vi "MoD Main-Optimize - HPLC - SUZUKI 04122017_ Simulate.vi"() -> ()   [LabVIEW 2015]
uses:
  <vilib>/ni845x/ni845x.llb/ni845xControl.ctl
  <vilib>/addons/control/pid/pid.llb/PID Control Input Filter (DBL).vi
  <vilib>/addons/control/pid/autopid.llb/PID Online Autotuning (Relay Feedback).vi
  <vilib>/addons/control/pid/NI_PID_autopid.lvlib
  <vilib>/addons/control/pid/NI_PID_pid.lvlib
  <vilib>/MakerHub/LINX/LMH-LINX.lvlib
  <vilib>/MakerHub/LINX/Public/Peripherals/Digital/Digital Write 1 Chan.vi
panel:
  out "Is current Exp a Redo?":bool=TRUE
  in  "Debug_run_button":bool
  out "Phase_Sensor_voltage":dbl
  out "P_tot":dbl
  out "pause for ms":bool=TRUE
  out "stop_xl_write":bool=TRUE
  out "Num_exp_till_pause":i32
  out "Syringe_pump?":bool=TRUE
  out "System Error":bool=TRUE
  out "error out":errorcluster
  out "Pump setpoint(ul/min) 6":dbl format="%#_13g"
  out "Pump setpoint(ul/min) 5":dbl format="%#_13g"
  out "Pump setpoint(ul/min) 4":dbl format="%#_13g"
  out "Pump setpoint(ul/min) 3":dbl format="%#_13g"
  out "Pump setpoint(ul/min) 2":dbl format="%#_13g"
  out "Pump setpoint(ul/min) 1":dbl format="%#_13g"
  out "Volume (ul) 5":dbl format="%#_13g"
  out "Volume (ul) 4":dbl format="%#_13g"
  out "Volume (ul) 3":dbl format="%#_13g"
  out "Volume (ul) 2":dbl format="%#_13g"
  out "Volume (ul) 1":dbl format="%#_13g"
  in  "tau 5":dbl format="%#_13g"
  out "tau 4":dbl format="%#_13g"
  out "tau 3":dbl format="%#_13g"
  out "tau 2":dbl format="%#_13g"
  out "tau 1":dbl format="%#_13g"
  out "Reactor Length":dbl format="%#_13g"
  out "Flowrate Sensor 2":dbl format="%#_13g"
  out "Flowrate Sensor 1":dbl format="%#_13g"
  out "Pressure 2":dbl format="%#_13g"
  out "Pressure 1":dbl format="%#_13g"
  out "Temperature Control 5":bool=TRUE
  out "Temperature Control 4":bool=TRUE
  out "Temperature Control 3":bool=TRUE
  out "Temperature Control 2":bool=TRUE
  out "Temperature Control 1":bool=TRUE
  out "Temperature SP 5":dbl format="%#_g'C"
  out "Temperature SP 4":dbl format="%#_g'C"
  out "Temperature SP 3":dbl format="%#_g'C"
  out "Temperature SP 2":dbl format="%#_g'C"
  out "Temperature SP 1":dbl format="%#_g'C"
  in  "Bay Temperature 5":dbl
  in  "SSR Duration 5":dbl
  in  "SSR Duration 4":dbl
  in  "SSR Duration 3":dbl
  in  "SSR Duration 2":dbl
  in  "SSR Duration 1":dbl
  in  "Total Product Amount":dbl=1.0 format="%#_gml"
  out "Setup Error":bool=TRUE
  out "Error Message":string
  out "ID CTR":i32
  in  "Tab Control 2":enum32{"Faults", "Devices"}(tab)=enum."Devices"
  out "Fault Cluster":T1
  in  "COMM Port:: Harvard Syringe Pump":refnum<visa-resource-name>="COM5"
  in  "Sample Valve COMM::Port":refnum<visa-resource-name>="COM6"
  in  "Arduino COMM Port":refnum<visa-resource-name>="COM3"
  in  "COMM Port :: Milligat Pumps":refnum<visa-resource-name>="COM10"
  in  "IR Sensor Device":T2="USB0::0x3923::0x7514::01B3FF21::RAW"
  in  "Tab Control":enum32{"Setup", "Parameters", "Monitoring"}(tab)
  in  "System decide help Button":bool
  in  "Reaction Scheme Confirm":bool
  in  "Synthesis Route Array":string[](array[string])=["3-Br-Pyridine _ Biphenyl", "K2CO3", "PhB(OH)2", "", "", ""]
  in  "Manual/Automated":bool
  in  "Save Button":bool
  in  "Open Button":bool
  in  "New rxn scheme button":bool
  in  "System decide help Button 2":bool
  out "Setup Confirm":bool=TRUE
  in  "BAY 1":u16(ring) items=["                 Bypass", "             Hot Reactor", "               Separator"]
  in  "BAY 5":u16(ring) items=["                     Bypass", "                Hot Reactor", "                 Separator"]
  in  "BAY 4":u16(ring) items=["                     Bypass", "                Hot Reactor", "                  Separator"]
  in  "BAY 3":u16(ring)=1 items=["                     Bypass", "                 Hot Reactor", "                  Separator"]
  in  "BAY 2":u16(ring) items=["                     Bypass", "                Hot Reactor", "                  Separator"]
  in  "System Parameters Help Button":bool
  in  "System Parameters Confirm Button":bool
  in  "Bay Parameters":T3={"Pump 1 Reagent Concentration"=0.8, "Pump 2 Reagent Concentration"=0.55, "Pump 3 Reagent Concentration"=0.4, "Pump 4 Reagent Concentration"=0.0, "Pump 5 Reagent Concentration"=0.0, "Bay 1 Parameters"={"Pump 1 Flowrate"=0.0, "optimize_temp"=FALSE, "optimize_tau"=TRUE, "Run at set flowrate"=FALSE, "Pump 2 Flowrate"=0.0, "Temperature Params"=[0.0, 40.0, 100.0], "pump params 1"=[0.0, 32.5, 325.0], "pump params 2"=[0.0, 32.5, 325.0]}, "Bay 2 Parameters"={"Pump 3 Flowrate"=0.0, "optimize_temp"=FALSE, "optimize_tau"=TRUE, "Run at set flowrate"=FALSE, "Temperature Params"=[0.0, 40.0, 100.0], "Resisdence time params"=[0.0, 65.0, 650.0], "pump_at_ratio"=FALSE, "pump_num_ratio"=0.0}, "Bay 3 Parameters"={"Pump 4 Flowrate"=0.0, "optimize_temp"=TRUE, "optimize_tau"=FALSE, "Run at set flowrate"=FALSE, "Temperature Params"=[0.0, 40.0, 100.0], "Resisdence time params"=[0.0, 0.0, 0.0], "pump_at_ratio"=FALSE, "pump_num_ratio"=0.0}, "Bay 4 Parameters"={"Pump 5 Flowrate"=40.0, "Run at set flowrate"=FALSE, "optimize_temp"=FALSE, "optimize_tau"=FALSE, "Resisdence time params"=[0.0, 36.0, 225.0], "Temperature Params"=[0.0, 40.0, 80.0], "pump_at_ratio"=FALSE, "pump_num_ratio"=0.0}, "Bay 5 Parameters"={"Pump 6 Flowrate"=0.0, "Run at set flowrate"=FALSE, "optimize_temp"=FALSE, "optimize_tau"=FALSE, "Resisdence time params"=[0.0, 0.0, 0.0], "Temperature Params"=[0.0, 0.0, 0.0], "pump_at_ratio"=FALSE, "pump_num_ratio"=0.2}, "Bay 1 Flow Rate Ratio \n(Pump 1: Pump 2)"=1.0, "tube_id(in)"=[enum.".02", enum.".03", enum.".03", enum.".03", enum.".03"], "xml_filename"="temp_xml", "Excel File Name"="C:\\Users\\HPLC\\Dropbox (MIT)\\MoD Files\\Data\\HWE Results\\SUZUKI Optimization HPLC - 04122017", "hplc File Name"="C:\\Chem32\\1\\Data\\MOD", "Matlab File"="C:\\Users\\HPLC\\Dropbox (MIT)\\MoD Files\\Data\\SUZUKI 04132017b", "Syringe for Pump 2?"=FALSE, "Num_conditons_per_wait"=1.0, "Continue from previous optimization?"=FALSE, "Pump 6 Reagent Concentration"=0.0, "Pause before analysis?"=FALSE, "Hplc Wait time(min)"=0.04} {"Hplc Wait time(min)" format="%#_13g"; "Pump 6 Reagent Concentration" format="%#_6gM"; "Bay 5 Parameters"."Temperature Params" format="%#_g'C"; "Bay 4 Parameters"."Temperature Params" format="%#_g'C"; "Bay 3 Parameters"."Temperature Params" format="%#_g'C"; "Bay 2 Parameters"."Temperature Params" format="%#_g'C"; "Bay 1 Parameters"."Temperature Params" format="%#_g'C"; "Pump 5 Reagent Concentration" format="%#_6gM"; "Pump 4 Reagent Concentration" format="%#_6gM"; "Pump 3 Reagent Concentration" format="%#_6gM"; "Pump 2 Reagent Concentration" format="%#_6gM"; "Pump 1 Reagent Concentration" format="%#_6gM"}
  out "System Confirm Not Clicked":string
  out "Setup Confirm 2":bool=TRUE
  out "Current Experiment":dbl
  in  "Total Number of Experiments":dbl=33.0
  out "Phase Sensor Chart":T4(graph)
  out "HPLC Analysis":bool
  out "Equlibrating Temperature":bool
  out "Flushing System":bool
  out "Calculate condition":bool
  out "System Flush Wait Time":u8(slide) scale=0.0..1149.042355163602
  out "Temperature 5":dbl format="%#_g'C"
  out "Temperature 4":dbl format="%#_g'C"
  out "Temperature 3":dbl format="%#_g'C"
  out "Temperature 2":dbl format="%#_g'C"
  out "Temperature 1":dbl format="%#_g'C"
  out "Flowrate Chart":T5(graph)
  out "Bay 5":u16(ring) items=["                     Bypass", "                   Reactor1", "               Separator"]
  out "Bay 4":u16(ring) items=["                     Bypass", "                   Reactor1", "               Separator"]
  out "Bay 3":u16(ring) items=["                     Bypass", "                   Reactor1", "               Separator"]
  out "Bay 2":u16(ring) items=["                     Bypass", "                   Reactor1", "               Separator"]
  out "Bay 1":u16(ring) items=["                     Bypass", "                   Reactor1", "               Separator"]
  out "Teperature Chart":T5(graph)
  out "Pump Setpoints Chart":T5(graph)
  out "Pressure Chart":T5(graph)
  out "Optimization_loop_index":i32
  out "curr_wait_time":dbl
  out "total_flush_time":dbl
  out "Temp SS? 5":bool=TRUE
  out "Temp SS? 4":bool=TRUE
  out "Temp SS? 3":bool=TRUE
  out "Temp SS? 2":bool=TRUE
  out "Temp SS? 1":bool=TRUE
  out "System Flushed?":bool
  out "stop_button clicked":bool
  out "Total System Resisdence Time(min)":dbl
  out "Will Redo Next Exp?":bool=TRUE
  out "Stop":bool=TRUE
  in  "Run_Stop_cluster":T6
  # "Molecules on Demand"
  # "Synthesis Route"
  # "Reagent List"
  # "1"
  # "2"
  # "1"
  # "3"
  # "2"
  # "4"
  # "3"
  # "5"
  # "4"
  # "6"
  # "5"
  # "Product"
  # "6"
  # "Have system decide based on synthesis route"
  # "Manually enter bay configuration"
  # "System Schematic"
  # "Optimization Parameters"
  # "Bay"
  # "Tube ID (in)"
  # "1."
  # "2."
  # "3."
  # "4."
  # "5."
  # "Pause after"
  # "Experiments"
  # "Reporting"
  # "XML Output File Name"
  # "Excel Output File Name"
  # "HPLC File Path"
  # "MATLAB File Path"
  # "Temperature"
  # "Flowrate(ul/min)"
  # "Setpoint"
  # "Lower Bound"
  # "Upper Bound"
  # "Optimize?"
  # "-or-"
  # "Run at"
  # "times incoming flow"
  # "Temperature"
  # "Flowrate(ul/min)"
  # "Setpoint"
  # "Lower Bound"
  # "Upper Bound"
  # "Optimize?"
  # "-or-"
  # "Run at"
  # "times incoming flow"
  # "Temperature"
  # "Flowrate(ul/min)"
  # "Setpoint"
  # "Lower Bound"
  # "Upper Bound"
  # "Optimize?"
  # "-or-"
  # "Run at"
  # "times incoming flow"
  # "Temperature"
  # "Flowrate 3 (ul/min)"
  # "Setpoint"
  # "Lower Bound"
  # "Upper Bound"
  # "Optimize?"
  # "-or-"
  # "Run at"
  # "times incoming flow"
  # "Temperature"
  # "Flowrate 1(ul/min)"
  # "Flowrate 2(ul/min)"
  # "Setpoint"
  # "Lower Bound"
  # "Upper Bound"
  # "Optimize?"
  # "Temperature('C)"
  # "Pressure (psi)"
  # "Flowrate (ul/min)"
  # "Pump Flowrate Setpoints(ul/min)"
  # "Phase Sensor Value"
  # "Experimental Steps"
  # "Calculated new conditions"
  # "Flushed System"
  # "Analyzed HPLC"
  # "Equilibrated Temperature"
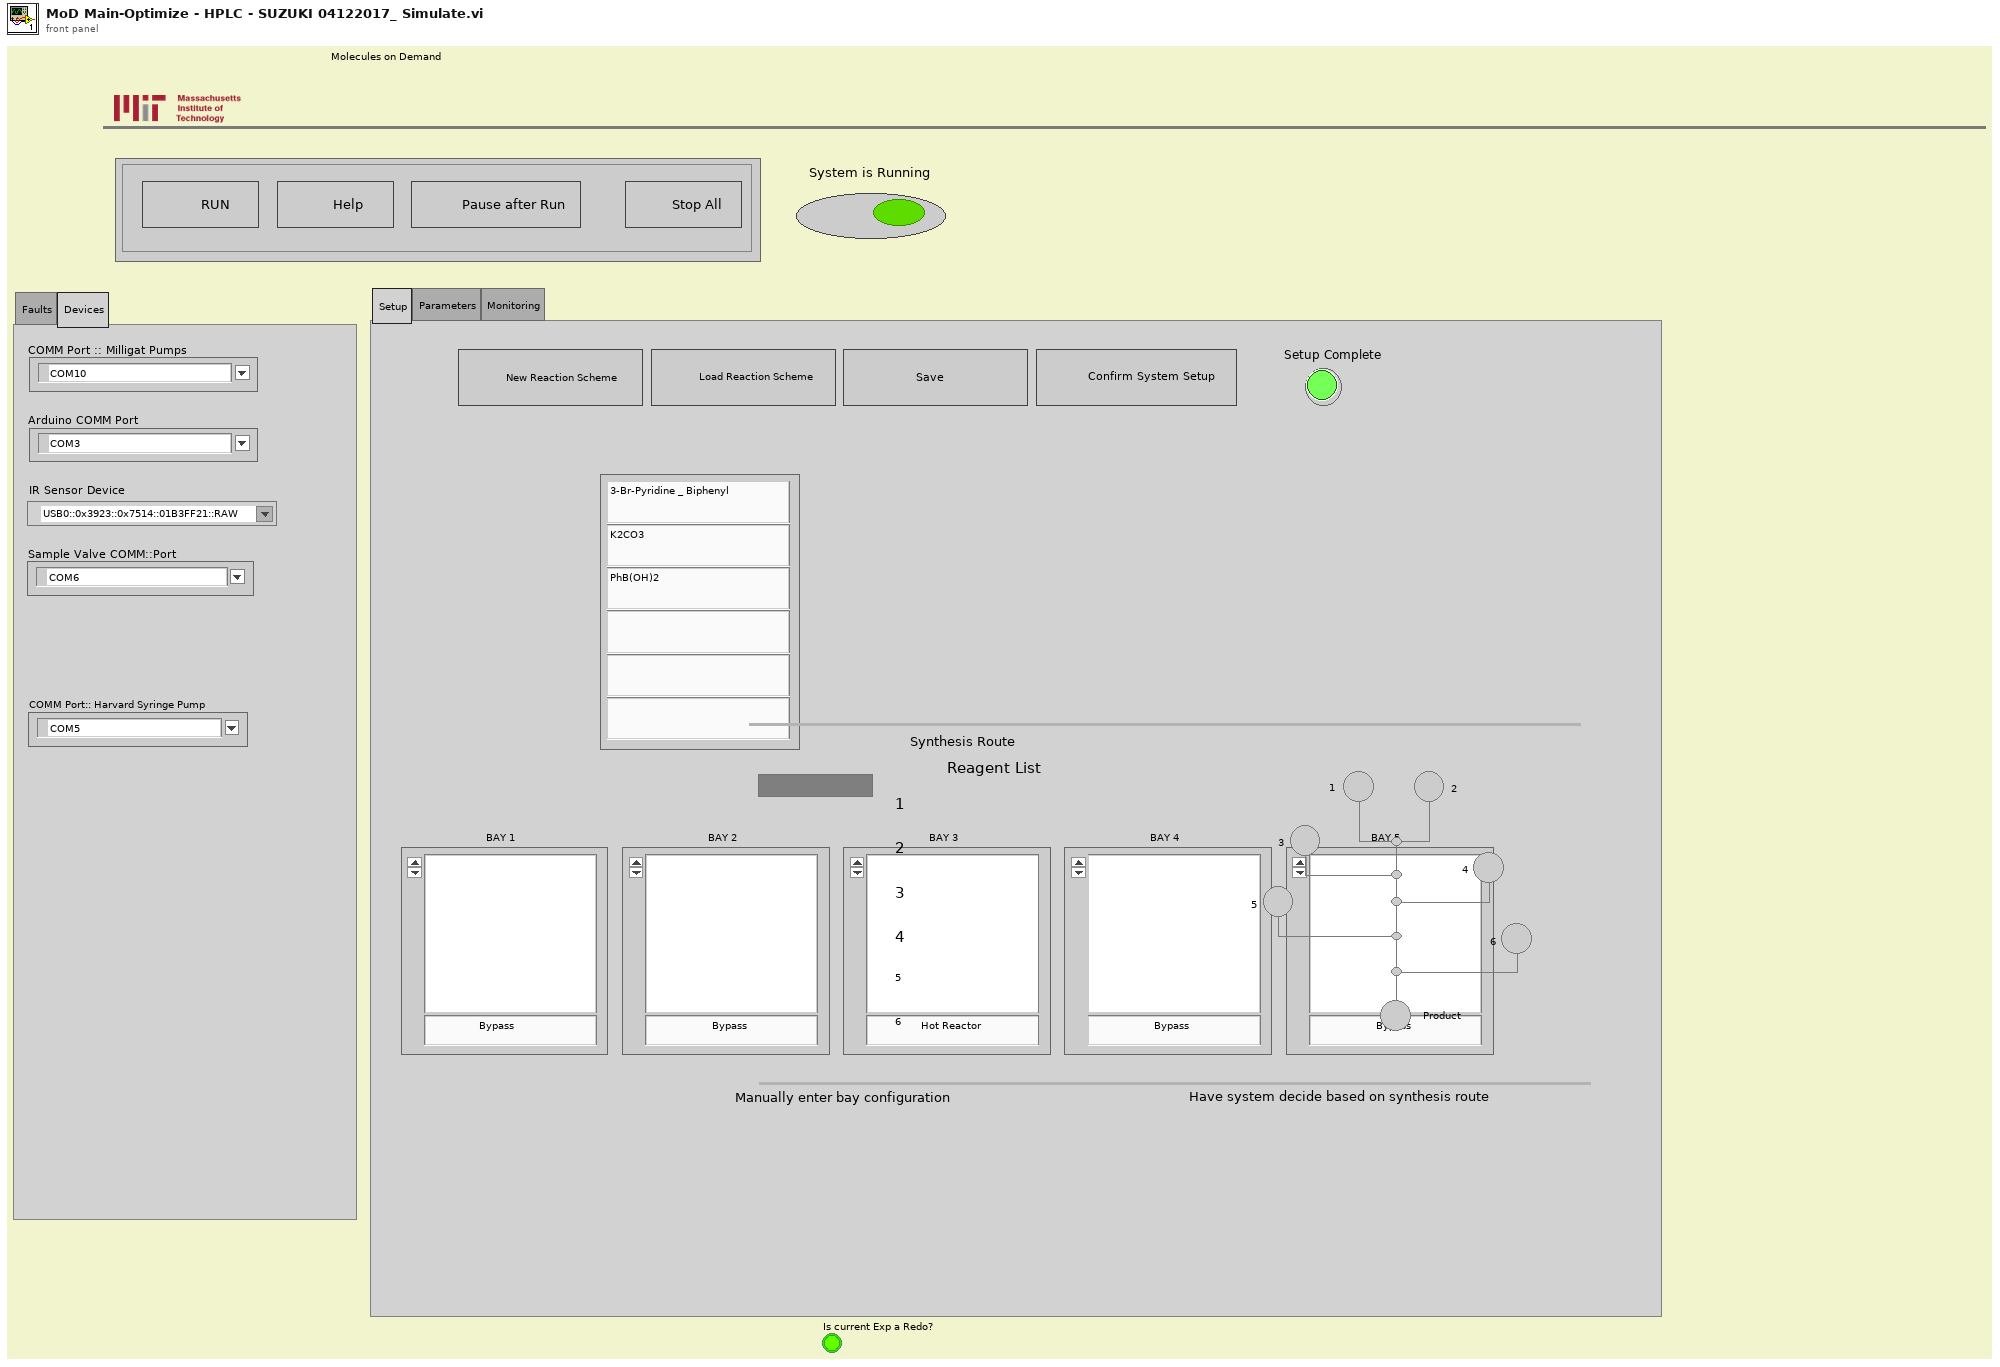
[diagram p1: front panel]
types:
  T1 = cluster{"Pump COMM Port":bool, "Pressure":bool, "Flow Rate":bool, "Temperature Sensor COMM Port":bool, "Arduino COMM Port":bool, "Chiller COMM Port":bool}
  T2 = typedef "ni845xControl.ctl" = refnum<k21>
  T3 = cluster{"Pump 1 Reagent Concentration":dbl, "Pump 2 Reagent Concentration":dbl, "Pump 3 Reagent Concentration":dbl, "Pump 4 Reagent Concentration":dbl, "Pump 5 Reagent Concentration":dbl, "Bay 1 Parameters":cluster{"Pump 1 Flowrate":dbl, "optimize_temp":bool, "optimize_tau":bool, "Run at set flowrate":bool, "Pump 2 Flowrate":dbl, "Temperature Params":dbl[], "pump params 1":dbl[], "pump params 2":dbl[]}, "Bay 2 Parameters":cluster{"Pump 3 Flowrate":dbl, "optimize_temp":bool, "optimize_tau":bool, "Run at set flowrate":bool, "Temperature Params":dbl[], "Resisdence time params":dbl[], "pump_at_ratio":bool, "pump_num_ratio":dbl}, "Bay 3 Parameters":cluster{"Pump 4 Flowrate":dbl, "optimize_temp":bool, "optimize_tau":bool, "Run at set flowrate":bool, "Temperature Params":dbl[], "Resisdence time params":dbl[], "pump_at_ratio":bool, "pump_num_ratio":dbl}, "Bay 4 Parameters":cluster{"Pump 5 Flowrate":dbl, "Run at set flowrate":bool, "optimize_temp":bool, "optimize_tau":bool, "Resisdence time params":dbl[], "Temperature Params":dbl[], "pump_at_ratio":bool, "pump_num_ratio":dbl}, "Bay 5 Parameters":cluster{"Pump 6 Flowrate":dbl, "Run at set flowrate":bool, "optimize_temp":bool, "optimize_tau":bool, "Resisdence time params":dbl[], "Temperature Params":dbl[], "pump_at_ratio":bool, "pump_num_ratio":dbl}, "Bay 1 Flow Rate Ratio \n(Pump 1: Pump 2)":dbl, "tube_id(in)":enum16{".01", ".02", ".03", ".04"}[], "xml_filename":string, "Excel File Name":string, "hplc File Name":string, "Matlab File":string, "Syringe for Pump 2?":bool, "Num_conditons_per_wait":dbl, "Continue from previous optimization?":bool, "Pump 6 Reagent Concentration":dbl, "Pause before analysis?":bool, "Hplc Wait time(min)":dbl}
  T4 = cluster{"[0]":i32, "[1]":i32, "[2]":i32, "[3]":i32, "[4]":i32, "[5]":i32, "[6]":i32, "[7]":i32, "[8]":i32}
  T5 = cluster{"[0]":dbl, "[1]":dbl, "[2]":dbl, "[3]":dbl, "[4]":dbl, "[5]":dbl, "[6]":dbl, "[7]":dbl, "[8]":dbl}
  T6 = cluster{"Stop":bool, "Help Button":bool, "Run":bool, "Stop Run Button":bool}
  T7 = cluster{"Proportional gain Kc":dbl, "Integral time Ti (sec)":dbl, "Derivative time Ti (sec)":dbl}
  T8 = cluster{"type of controller":enum16{"P", "PI", "PID"}, "relay cycles":i32, "relay amplitude":dbl, "control specifications":enum16{"Fast", "Normal", "Slow"}, "PV noise level":dbl}
  T9 = cluster{"proportional gain (Kc)":dbl, "integral time (Ti, min)":dbl, "derivative time (Td, min)":dbl}
  T10 = typedef "LMH-LINX.lvlib/LINX Ref.ctl" = cluster{"IO":T11, "Interface":T12, "LINX Device Config":T13}
  T11 = typedef "LMH-LINX.lvlib/Platform.ctl" = enum16{"Remote", "Local"}
  T12 = typedef "LMH-LINX.lvlib/Interface.ctl" = enum16{"Serial", "TCP"}
  T13 = typedef "LMH-LINX.lvlib/Device.lvlib/LINX Device Config.ctl" = cluster{"Interface":T12, "COM Port":refnum<visa-resource-name>, "TCP Configuration":T14, "Device Family":u8, "Device ID":u8, "Device Name":string, "TCP Ref":refnum<k5>, "Channels":T15}
  T14 = typedef "LMH-LINX.lvlib/Device.lvlib/TCP Config.ctl" = cluster{"IP Address":string, "Port":u16}
  T15 = typedef "LMH-LINX.lvlib/Channels.ctl" = cluster{"DI":u8[], "DO":u8[], "AI":u8[], "AO":u8[], "PWM":u8[], "QE":u8[], "UART":u8[], "I2C 2":u8[], "SPI":u8[], "CAN":u8[], "Servo":u8[], "AI Ref (V)":dbl, "AI Resolution (Bits)":u8, "AO Ref (V)":dbl, "AO Resolution (Bits)":u8}
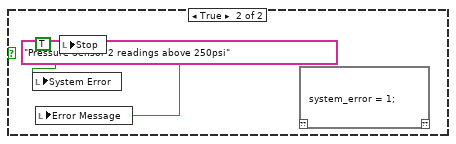
[diagram p2: hidden frame]
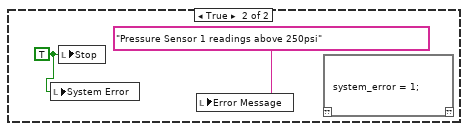
[diagram p3: hidden frame]
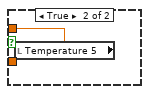
[diagram p4: hidden frame]
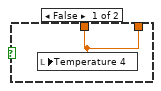
[diagram p5: hidden frame]
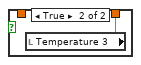
[diagram p6: hidden frame]
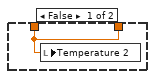
[diagram p7: hidden frame]
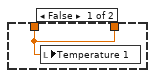
[diagram p8: hidden frame]
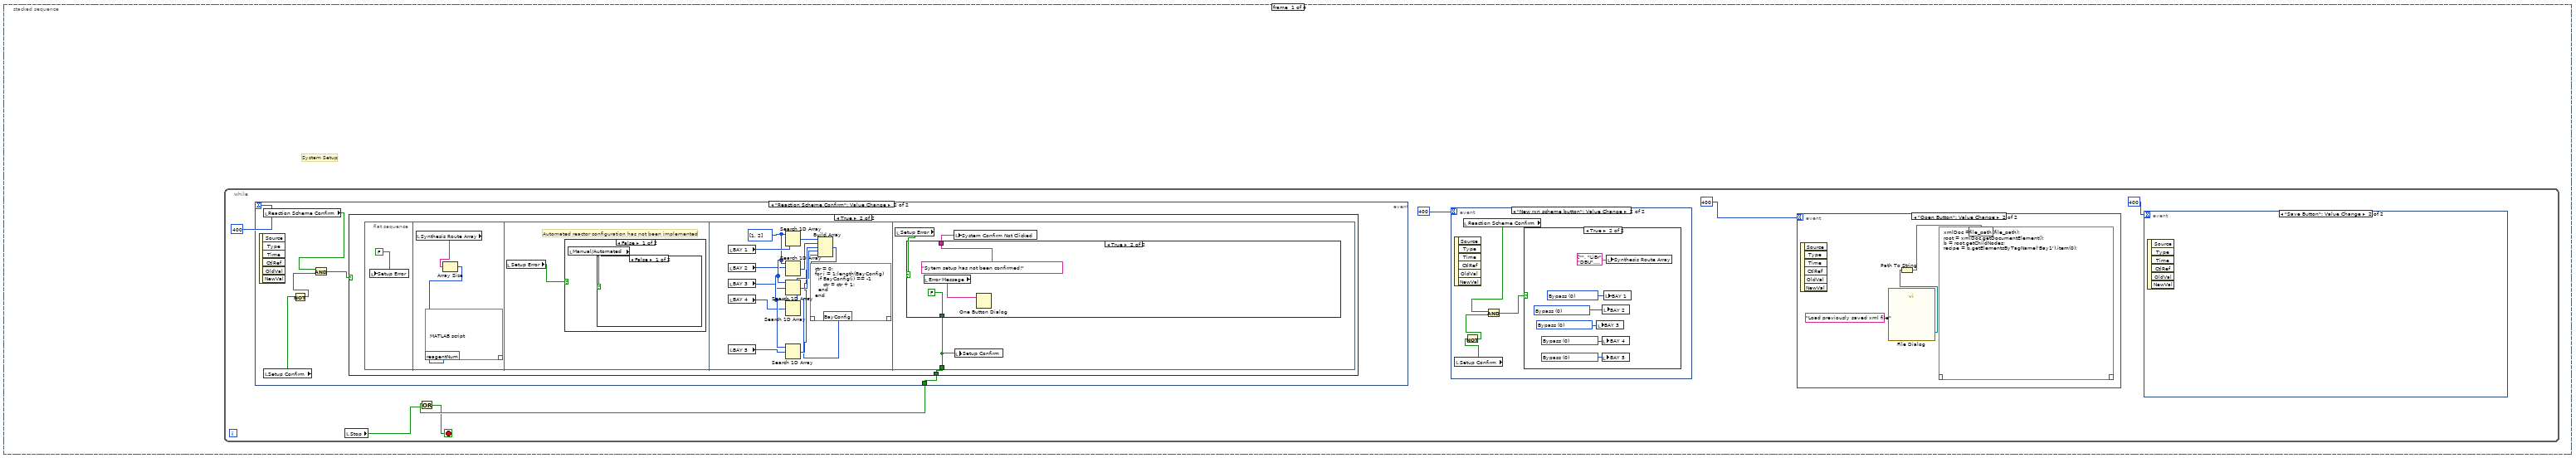
[diagram p9: hidden frame]
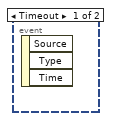
[diagram p10: hidden frame]
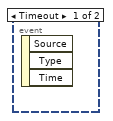
[diagram p11: hidden frame]
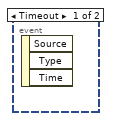
[diagram p12: hidden frame]
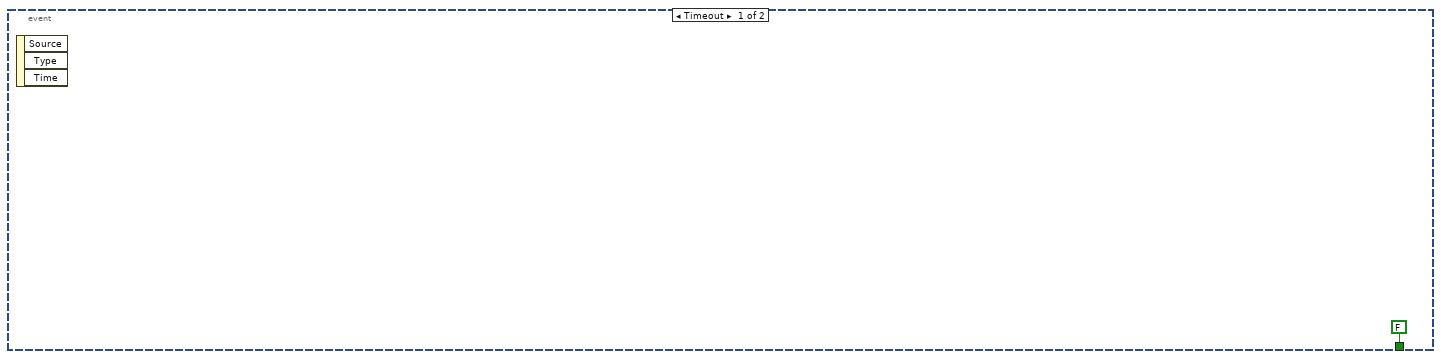
[diagram p14: hidden frame]
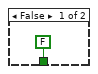
[diagram p15: hidden frame]
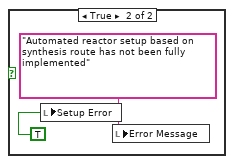
[diagram p16: hidden frame]
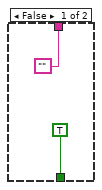
[diagram p18: hidden frame]
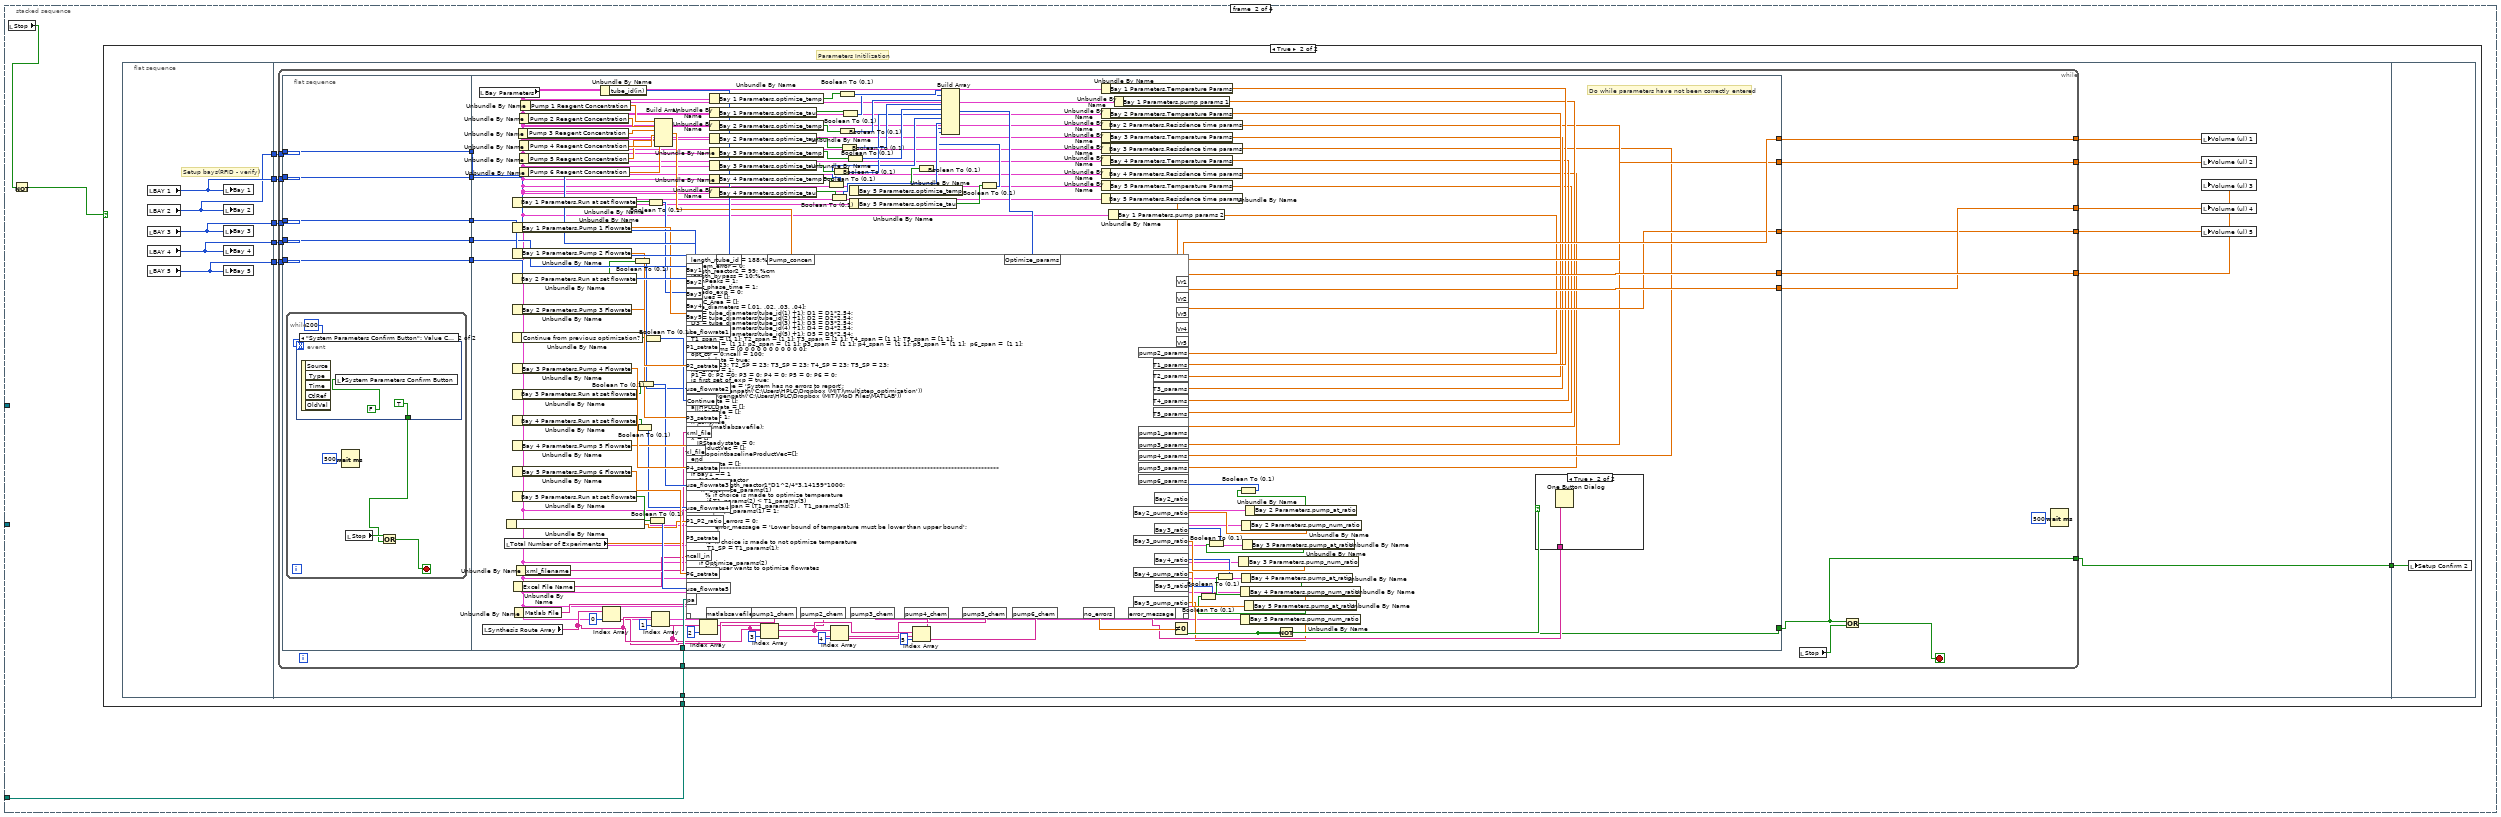
[diagram p19: hidden frame]
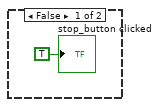
[diagram p20: hidden frame]
diagram:
  # "Assume User always uses the first bay first"
  n1 = flat-sequence {
    tunnel: ["COMM Port :: Milligat Pumps"] -> w6
    tunnel: ["Arduino COMM Port"] -> w5
    tunnel: ["COMM Port:: Harvard Syringe Pump"] -> w2
    tunnel: ["Bay Parameters"] -> w1
    tunnel: [w44] -> w7
    tunnel: w6 -> [w44]
    tunnel: w5 -> [_]
    tunnel: [w27] -> w4
    tunnel: [w25] -> w3
    tunnel: w2 -> [w25]
    tunnel: w1 -> [w23]
    tunnel: w7 -> [w48]
    tunnel: w4 -> [w47]
    tunnel: w3 -> [w45]
    frame #0 {
      w11 = FALSE ("Equlibrating Temperature")
      n2 = script code="TempArr1=[23 23 23 23 23 23 23 23 23 23]';\nTempArr2=[23 23 23 23 23 23 23 23 23 23]';\nTempArr3=[23 23 23 23 23 23 23 23 23 23]';\nTempArr4=[23 23 23 23 23 23 23 23 23 23]';\nTempArr5=[23 23 23 23 23 23 23 23 23 23]';\ntemp_error1 =0;\ntemp_error2 =0;\ntemp_error3 =0;\ntemp_error4 =0;\ntemp_error5 =0;\ntemp_check1 = 0;\ntemp_check2 = 0;\ntemp_check3 = 0;\ntemp_check4 = 0;\ntemp_check5 = 0;\nT1=23;\nT2=23;\nT3=23;\nT4=23;\nT5=23;"() -> ()  [unwired: 1 in, 1 out]
      "Stop" <- FALSE ("Stop")
      "ID CTR" <- 0
      "Setup Confirm" <- FALSE ("Setup Confirm")
      "Setup Error" <- FALSE ("Setup Error")
      "Reactor Length" <- 10.5
      "System Error" <- FALSE ("System Error")
      "Num_exp_till_pause" <- 0 ("Num_exp_till_pause")
      "Equlibrating Temperature" <- w11
      "Calculate condition" <- w11
      "Flushing System" <- w11
      "HPLC Analysis" <- w11
      "Setup Confirm 2" <- FALSE ("Setup Confirm 2")
      "stop_xl_write" <- FALSE ("stop_xl_write")
    }
    frame #1 {
      w38 = 23
      (unwired) path "C:/Users/User1/Documents/Lab/MoD/Images"
      n3 = local write "Debug_run_button"(TRUE) -> ()
      n4 = local read "BAY 2"() -> (w42:u16)
      n5 = local read "BAY 3"() -> (w41:u16)
      n6 = local read "BAY 4"() -> (w40:u16)
      n7 = local read "BAY 5"() -> (w39:u16)
      n8 = local read "BAY 1"() -> (w43:u16)
      n9 = local write "Bay 1"(w43) -> ()
      n10 = local write "Bay 2"(w42) -> ()
      n11 = local write "Bay 3"(w41) -> ()
      n12 = local write "Bay 4"(w40) -> ()
      n13 = local write "BAY 5"(w39) -> ()
      n14 = Unbundle By Name(w23) -> ("Syringe for Pump 2?"=→"Syringe_pump?":bool)
      n15 = local write "Temperature 1"(w38) -> ()
      n16 = local write "Temperature 2"(w38) -> ()
      n17 = local write "Temperature 3"(w38) -> ()
      n18 = local write "Temperature 4"(w38) -> ()
      n19 = local write "Temperature 5"(w38) -> ()
      n20 = local write "Temperature SP 1"(w38) -> ()
      n21 = local write "Temperature SP 2"(w38) -> ()
      n22 = local write "Temperature SP 3"(w38) -> ()
      n23 = local write "Temperature SP 4"(w38) -> ()
      n24 = local write "Temperature SP 5"(w38) -> ()
      n25 = Unbundle By Name(w23) -> ("Pause before analysis?"=→"pause for ms":bool)
      n26 = Current VI's Path() -> (path=w31:path)
      n27 = Strip Path(path=w31) -> (stripped path=w29:path)  [unwired: 1 out]
      n28 = Strip Path(path=w29) -> (stripped path=w28:path)  [unwired: 1 out]
      n29 = Build Path(base path=w28, name or relative path="MATLAB") -> (appended path=w27:path)
      "Pump setpoint(ul/min) 1" <- 0.0 ("Pump setpoint(ul/min) 1")
      "Pump setpoint(ul/min) 2" <- 0.0 ("Pump setpoint(ul/min) 2")
      "Pump setpoint(ul/min) 3" <- 0.0 ("Pump setpoint(ul/min) 3")
      "Pump setpoint(ul/min) 4" <- 0.0 ("Pump setpoint(ul/min) 4")
      "Pump setpoint(ul/min) 5" <- 0.0 ("Pump setpoint(ul/min) 5")
      "Pump setpoint(ul/min) 6" <- 0.0 ("Pump setpoint(ul/min) 6")
    }
    frame #2 {
      # "Main Help Dialog Popup"
      n30 = while {
        stop <- w989 stop-if-true
        n31 = event shown="[1] \"Run_Stop_cluster.Help Button\": Value Change" {
          selector: _ -> [_ _ _ _ _ _]
          dyn-events: _ -> [_ _ _ _ _ _]
          timeout: 100 -> [_ _ _ _ _ _]
          event Timeout {
            n32 = event-data() -> ()  [unwired: 1 in, 3 out]
          }
          event "Run_Stop_cluster.Help Button": Value Change {
            n33 = local read "Run_Stop_cluster"() -> (w992:T6)
            n34 = event-data() -> ()  [unwired: 1 in, 4 out]
            n35 = Unbundle By Name(w992) -> ("Help Button"=w991:bool)
            n36 = case shown="True" w991 {
              frame False {
              }
              frame True {
                n37 = call "help.vi"() -> ()  [unwired: 11 in]
              }
            }
          }
          event "System decide help Button": Value Change {
            n38 = event-data() -> ()  [unwired: 1 in, 5 out]
            n39 = call "help_synthesis_man-auto_instructions.vi"() -> ()  [unwired: 12 in]
          }
          event "System Parameters Help Button": Value Change {
            n40 = event-data() -> ()  [unwired: 1 in, 5 out]
            n41 = call "help_parameters_setup.vi"() -> ()  [unwired: 12 in]
          }
          event "System decide help Button 2": Value Change {
            n42 = event-data() -> ()  [unwired: 1 in, 5 out]
            n43 = call "help_synthesis_route_instructions.vi"() -> ()  [unwired: 12 in]
          }
          event "Run_Stop_cluster.Stop": Value Change {
            n44 = event-data() -> ()  [unwired: 1 in, 5 out]
            n45 = local write "Stop"(TRUE) -> ()
          }
        }
        n46 = local read "Stop"() -> (w989:bool)
      }
      n47 = stacked-sequence {
        tunnel: w48 -> [_ _ _ _]
        tunnel: w47 -> [_ w200 _ _]
        tunnel: w45 -> [_ _ _ w366]
        frame #0 {
          # "System Setup"
          n48 = while {
            stop <- w146 stop-if-true
            n49 = event shown="[1] \"Reaction Scheme Confirm\": Value Change" {
              selector: _ -> [_ _]
              dyn-events: _ -> [_ _]
              timeout: 400 -> [_ _]
              tunnel: [FALSE w164] -> w148
              event Timeout {
                n50 = event-data() -> ()  [unwired: 1 in, 3 out]
              }
              event "Reaction Scheme Confirm": Value Change {
                n51 = event-data() -> ()  [unwired: 1 in, 6 out]
                n52 = local read "Reaction Scheme Confirm"() -> (w168:bool)
                n53 = local read "Setup Confirm"() -> (w166:bool)
                n54 = Not(x=w166) -> (.not. x?=w165:bool)
                n55 = And(x=w168, y=w165) -> (x .and. y?=w167:bool)
                n56 = case shown="True" w167 {
                  tunnel: [FALSE w170] -> w164
                  frame False {
                  }
                  frame True {
                    n57 = flat-sequence {
                      tunnel: [w190] -> w170
                      frame #0 {
                        n58 = local write "Setup Error"(FALSE) -> ()
                      }
                      frame #1 {
                        n59 = local read "Synthesis Route Array"() -> (w173:string[])
                        n60 = Array Size(array=w173) -> (size(s)=w172:i32)
                        n61 = script code="MATLAB script"("reagentNum"=w172) -> ()  [unwired: 1 in, 1 out]
                      }
                      frame #2 {
                        # "Automated reactor configuration has not been implemented"
                        n62 = local read "Setup Error"() -> (w174:bool)
                        n63 = case shown="False" w174 {
                          frame False {
                            n64 = local read "Manual/Automated"() -> (w175:bool)
                            n65 = case shown="False" w175 {
                              frame False {
                              }
                              frame True {
                                n66 = local write "Setup Error"(TRUE ("Setup Error")) -> ()
                                n67 = local write "Error Message"("Automated reactor setup based on synthesis route has not been fully implemented") -> ()
                              }
                            }
                          }
                          frame True {
                          }
                        }
                      }
                      frame #3 {
                        w188 = i32[] [1, 2]
                        n68 = local read "BAY 1"() -> (w189:u16)
                        n69 = local read "BAY 2"() -> (w187:u16)
                        n70 = local read "BAY 3"() -> (w186:u16)
                        n71 = local read "BAY 4"() -> (w185:u16)
                        n72 = local read "BAY 5"() -> (w184:u16)
                        n73 = Search 1D Array(1D array=w188, element=w189) -> (index of element=w183:i32)  [unwired: 1 in]
                        n74 = Search 1D Array(1D array=w188, element=w187) -> (index of element=w182:i32)  [unwired: 1 in]
                        n75 = Search 1D Array(1D array=w188, element=w186) -> (index of element=w181:i32)  [unwired: 1 in]
                        n76 = Search 1D Array(1D array=w188, element=w185) -> (index of element=w180:i32)  [unwired: 1 in]
                        n77 = Search 1D Array(1D array=w188, element=w184) -> (index of element=w179:i32)  [unwired: 1 in]
                        n78 = Build Array(w183, w182, w181, w180, w179) -> (w178:i32[])
                        n79 = script code="ctr = 0;\nfor i = 1:length(BayConfig)\n  if BayConfig(i) == -1\n     ctr = ctr + 1;\n  end\nend"("BayConfig"=w178) -> ()  [unwired: 1 in, 1 out]
                      }
                      frame #4 {
                        n80 = local read "Setup Error"() -> (w192:bool)
                        n81 = case shown="True" w192 {
                          tunnel: [TRUE FALSE] -> w190
                          tunnel: ["" "Sytem setup has not been confirmed!"] -> w191
                          frame False {
                          }
                          frame True {
                            n82 = local read "Error Message"() -> (w197:string)
                            n83 = One Button Dialog(message=w197) -> ()  [unwired: 1 in, 1 out]
                          }
                        }
                        n84 = local write "System Confirm Not Clicked"(w191) -> ()
                        n85 = local write "Setup Confirm"(w190) -> ()
                      }
                    }
                  }
                }
              }
            }
            n86 = local read "Stop"() -> (w147:bool)
            n87 = Or(x=w148, y=w147) -> (x .or. y?=w146:bool)
            n88 = event shown="[1] \"New rxn scheme button\": Value Change" {
              selector: _ -> [_ _]
              dyn-events: _ -> [_ _]
              timeout: 400 -> [_ _]
              event Timeout {
                n89 = event-data() -> ()  [unwired: 1 in, 3 out]
              }
              event "New rxn scheme button": Value Change {
                n90 = event-data() -> ()  [unwired: 1 in, 6 out]
                n91 = local read "Setup Confirm"() -> (w153:bool)
                n92 = local read "Reaction Scheme Confirm"() -> (w154:bool)
                n93 = Not(x=w153) -> (.not. x?=w156:bool)
                n94 = And(x=w154, y=w156) -> (x .and. y?=w155:bool)
                n95 = case shown="True" w155 {
                  frame False {
                  }
                  frame True {
                    w157 = u16 0 items=["                     Bypass", "                Hot Reactor", "                 Separator"] ("BAY 5")
                    w158 = u16 0 items=["                     Bypass", "                Hot Reactor", "                  Separator"] ("BAY 4")
                    w159 = u16 0 items=["                     Bypass", "                 Hot Reactor", "                  Separator"] ("BAY 3")
                    w160 = u16 0 items=["                     Bypass", "                Hot Reactor", "                  Separator"] ("BAY 2")
                    w161 = u16 0 items=["                 Bypass", "             Hot Reactor", "               Separator"] ("BAY 1")
                    n96 = local write "BAY 3"(w159) -> ()
                    n97 = local write "BAY 4"(w158) -> ()
                    n98 = local write "BAY 5"(w157) -> ()
                    n99 = local write "BAY 2"(w160) -> ()
                    n100 = local write "BAY 1"(w161) -> ()
                    n101 = local write "Synthesis Route Array"(string[] ["", "LiBr", "DBU", "Aldehyde", "Water", "Toluene"] ("Synthesis Route Array")) -> ()
                  }
                }
              }
            }
            n102 = event shown="[1] \"Open Button\": Value Change" {
              selector: _ -> [_ _]
              dyn-events: _ -> [_ _]
              timeout: 400 -> [_ _]
              event Timeout {
                n103 = event-data() -> ()  [unwired: 1 in, 3 out]
              }
              event "Open Button": Value Change {
                n104 = event-data() -> ()  [unwired: 1 in, 6 out]
                n105 = call "File Dialog"("prompt"="Load previously saved xml file") -> ("selected path"=w151:path)  [unwired: 11 in, 3 out]
                n106 = Path To String(path=w151) -> (string=w150:string)
                n107 = script code="xmlDoc = xmlread(file_path);\nroot = xmlDoc.getDocumentElement();\nb = root.getChildNodes;\nrecipe = b.getElementsByTagName('Bay1').item(0);"("file_path"=w150) -> ()  [unwired: 1 in, 1 out]
              }
            }
            n108 = event shown="[1] \"Save Button\": Value Change" {
              selector: _ -> [_ _]
              dyn-events: _ -> [_ _]
              timeout: 400 -> [_ _]
              event Timeout {
                n109 = event-data() -> ()  [unwired: 1 in, 3 out]
              }
              event "Save Button": Value Change {
                n110 = event-data() -> ()  [unwired: 1 in, 6 out]
              }
            }
          }
        }
        frame #1 {
          n111 = local read "Stop"() -> (w199:bool)
          n112 = Not(x=w199) -> (.not. x?=w198:bool)
          n113 = case shown="True" w198 {
            tunnel: w200 -> [_ w203]
            frame False {
              "stop_button clicked" <- TRUE ("stop_button clicked")
            }
            frame True {
              # "Parameters Initilization"
              n114 = flat-sequence {
                tunnel: [w213] -> w208
                tunnel: [w212] -> w207
                tunnel: [w211] -> w206
                tunnel: [w210] -> w205
                tunnel: [w209] -> w204
                tunnel: w208 -> [w225]
                tunnel: w207 -> [w224]
                tunnel: w206 -> [w223]
                tunnel: w205 -> [w222]
                tunnel: w204 -> [w221]
                tunnel: w203 -> [w215]
                tunnel: [w214] -> w202
                tunnel: w202 -> [w364]
                frame #0 {
                  # "Setup bays(RFID - verify)"
                  n115 = local read "BAY 1"() -> (w213:u16)
                  n116 = local read "BAY 2"() -> (w212:u16)
                  n117 = local read "BAY 3"() -> (w211:u16)
                  n118 = local read "BAY 4"() -> (w210:u16)
                  n119 = local read "BAY 5"() -> (w209:u16)
                  n120 = local write "Bay 1"(w213) -> ()
                  n121 = local write "Bay 2"(w212) -> ()
                  n122 = local write "Bay 3"(w211) -> ()
                  n123 = local write "Bay 4"(w210) -> ()
                  n124 = local write "Bay 5"(w209) -> ()
                }
                frame #1 {
                  n125 = while {
                    tunnel: w225 -> [w245]
                    tunnel: w224 -> [w244]
                    tunnel: w223 -> [w243]
                    tunnel: w222 -> [w242]
                    tunnel: w221 -> [w241]
                    tunnel: [w240] -> w220
                    tunnel: [w239] -> w219
                    tunnel: [w238] -> w218
                    tunnel: [w237] -> w217
                    tunnel: [w236] -> w216
                    tunnel: w215 -> [w227]
                    tunnel: [w226] -> w214
                    stop <- w235 stop-if-true
                    n126 = flat-sequence {
                      tunnel: w241 -> [w246]
                      tunnel: w242 -> [w247]
                      tunnel: w243 -> [w248]
                      tunnel: w244 -> [w249]
                      tunnel: w245 -> [w250]
                      tunnel: [w250] -> w232
                      tunnel: [w249] -> w231
                      tunnel: [w248] -> w230
                      tunnel: [w247] -> w229
                      tunnel: [w246] -> w228
                      tunnel: [w350] -> w240
                      tunnel: [w349] -> w239
                      tunnel: [w348] -> w238
                      tunnel: [w347] -> w237
                      tunnel: [w346] -> w236
                      tunnel: [w302] -> w226
                      tunnel: w232 -> [w362]
                      tunnel: w231 -> [w361]
                      tunnel: w230 -> [w360]
                      tunnel: w229 -> [w359]
                      tunnel: w228 -> [w358]
                      tunnel: w227 -> [w298]
                      frame #0 {
                        n127 = while {
                          stop <- w254 stop-if-true
                          n128 = event shown="[1] \"System Parameters Confirm Button\": Value Change" {
                            selector: _ -> [_ _]
                            dyn-events: _ -> [_ _]
                            timeout: u32 200 ("milliseconds to wait") -> [_ _]
                            tunnel: [FALSE TRUE] -> w252
                            event Timeout {
                              n129 = event-data() -> ()  [unwired: 1 in, 3 out]
                            }
                            event "System Parameters Confirm Button": Value Change {
                              n130 = event-data() -> ()  [unwired: 1 in, 5 out]
                              n131 = local write "System Parameters Confirm Button"(FALSE) -> ()
                            }
                          }
                          n132 = Wait (ms)(milliseconds to wait=u32 500) -> ()  [unwired: 1 out]
                          n133 = local read "Stop"() -> (w255:bool)
                          n134 = Or(x=w255, y=w252) -> (x .or. y?=w254:bool)
                        }
                      }
                      frame #1 {
                        # "Do while parameters have not been correctly entered"
                        n135 = local read "Bay Parameters"() -> (w260:T3)
                        n136 = local read "Synthesis Route Array"() -> (w275:string[])
                        n137 = local read "Total Number of Experiments"() -> (w261:dbl)
                        n138 = Unbundle By Name(w260) -> ("Bay 1 Flow Rate Ratio \n(Pump 1: Pump 2)"=w301:dbl)
                        n139 = Unbundle By Name(w260) -> ("Continue from previous optimization?"=w297:bool)
                        n140 = Unbundle By Name(w260) -> ("Bay 1 Parameters.Run at set flowrate"=w345:bool)
                        n141 = Unbundle By Name(w260) -> ("Bay 1 Parameters.Pump 1 Flowrate"=w356:dbl)
                        n142 = Unbundle By Name(w260) -> ("Bay 1 Parameters.Pump 2 Flowrate"=w355:dbl)
                        n143 = Unbundle By Name(w260) -> ("Bay 2 Parameters.Run at set flowrate"=w343:bool)
                        n144 = Unbundle By Name(w260) -> ("Bay 2 Parameters.Pump 3 Flowrate"=w354:dbl)
                        n145 = Unbundle By Name(w260) -> ("Bay 3 Parameters.Pump 4 Flowrate"=w353:dbl)
                        n146 = Unbundle By Name(w260) -> ("Bay 3 Parameters.Run at set flowrate"=w342:bool)
                        n147 = Unbundle By Name(w260) -> ("Bay 4 Parameters.Run at set flowrate"=w339:bool)
                        n148 = Unbundle By Name(w260) -> ("Bay 4 Parameters.Pump 5 Flowrate"=w352:dbl)
                        n149 = Unbundle By Name(w260) -> ("Bay 5 Parameters.Pump 6 Flowrate"=w351:dbl)
                        n150 = Unbundle By Name(w260) -> ("Bay 5 Parameters.Run at set flowrate"=w338:bool)
                        n151 = Unbundle By Name(w260) -> ("Excel File Name"=w299:string)
                        n152 = Unbundle By Name(w260) -> ("Matlab File"=w295:string)
                        n153 = Unbundle By Name(w260) -> ("xml_filename"=w300:string)
                        n154 = Unbundle By Name(w260) -> ("Pump 3 Reagent Concentration"=w266:dbl)
                        n155 = Unbundle By Name(w260) -> ("Pump 2 Reagent Concentration"=w267:dbl)
                        n156 = Unbundle By Name(w260) -> ("Pump 4 Reagent Concentration"=w265:dbl)
                        n157 = Unbundle By Name(w260) -> ("Pump 5 Reagent Concentration"=w264:dbl)
                        n158 = Unbundle By Name(w260) -> ("Pump 6 Reagent Concentration"=w263:dbl)
                        n159 = Unbundle By Name(w260) -> ("Pump 1 Reagent Concentration"=w268:dbl)
                        n160 = Unbundle By Name(w260) -> ("tube_id(in)"=w357:enum16{".01", ".02", ".03", ".04"}[])
                        n161 = Index Array(array=w275, index=0) -> (element=w274:string)
                        n162 = Boolean To (0,1)(Boolean=w343) -> (0, 1=w294:i16)
                        n163 = Boolean To (0,1)(Boolean=w339) -> (0, 1=w340:i16)
                        n164 = Boolean To (0,1)(Boolean=w342) -> (0, 1=w341:i16)
                        n165 = Boolean To (0,1)(Boolean=w297) -> (0, 1=w296:i16)
                        n166 = Boolean To (0,1)(Boolean=w345) -> (0, 1=w344:i16)
                        n167 = Boolean To (0,1)(Boolean=w338) -> (0, 1=w337:i16)
                        n168 = Index Array(array=w275, index=1) -> (element=w269:string)
                        n169 = Build Array(w268, w267, w266, w265, w264, w263) -> (w262:dbl[])
                        n170 = Index Array(array=w275, index=2) -> (element=w270:string)
                        n171 = Unbundle By Name(w260) -> ("Bay 1 Parameters.optimize_temp"=w336:bool)
                        n172 = Unbundle By Name(w260) -> ("Bay 1 Parameters.optimize_tau"=w334:bool)
                        n173 = Unbundle By Name(w260) -> ("Bay 2 Parameters.optimize_temp"=w332:bool)
                        n174 = Unbundle By Name(w260) -> ("Bay 2 Parameters.optimize_tau"=w330:bool)
                        n175 = Unbundle By Name(w260) -> ("Bay 3 Parameters.optimize_temp"=w328:bool)
                        n176 = Unbundle By Name(w260) -> ("Bay 3 Parameters.optimize_tau"=w326:bool)
                        n177 = Unbundle By Name(w260) -> ("Bay 4 Parameters.optimize_temp"=w324:bool)
                        n178 = Unbundle By Name(w260) -> ("Bay 4 Parameters.optimize_tau"=w322:bool)
                        n179 = Index Array(array=w275, index=3) -> (element=w271:string)
                        n180 = Boolean To (0,1)(Boolean=w324) -> (0, 1=w323:i16)
                        n181 = Boolean To (0,1)(Boolean=w322) -> (0, 1=w321:i16)
                        n182 = Index Array(array=w275, index=4) -> (element=w272:string)
                        n183 = Boolean To (0,1)(Boolean=w326) -> (0, 1=w325:i16)
                        n184 = Boolean To (0,1)(Boolean=w332) -> (0, 1=w331:i16)
                        n185 = Boolean To (0,1)(Boolean=w336) -> (0, 1=w335:i16)
                        n186 = Boolean To (0,1)(Boolean=w330) -> (0, 1=w329:i16)
                        n187 = Boolean To (0,1)(Boolean=w334) -> (0, 1=w333:i16)
                        n188 = Boolean To (0,1)(Boolean=w328) -> (0, 1=w327:i16)
                        n189 = Unbundle By Name(w260) -> ("Bay 5 Parameters.optimize_temp"=w320:bool)
                        n190 = Unbundle By Name(w260) -> ("Bay 5 Parameters.optimize_tau"=w318:bool)
                        n191 = Index Array(array=w275, index=5) -> (element=w273:string)
                        n192 = Boolean To (0,1)(Boolean=w320) -> (0, 1=w319:i16)
                        n193 = Boolean To (0,1)(Boolean=w318) -> (0, 1=w317:i16)
                        n194 = Build Array(w335, w333, w331, w329, w327, w325, w323, w321, w319, w317) -> (w316:i16[])
                        n195 = Unbundle By Name(w260) -> ("Bay 1 Parameters.Temperature Params"=w313:dbl[])
                        n196 = Unbundle By Name(w260) -> ("Bay 2 Parameters.Temperature Params"=w312:dbl[])
                        n197 = Unbundle By Name(w260) -> ("Bay 2 Parameters.Resisdence time params"=w307:dbl[])
                        n198 = Unbundle By Name(w260) -> ("Bay 3 Parameters.Temperature Params"=w311:dbl[])
                        n199 = Unbundle By Name(w260) -> ("Bay 3 Parameters.Resisdence time params"=w306:dbl[])
                        n200 = Unbundle By Name(w260) -> ("Bay 4 Parameters.Temperature Params"=w310:dbl[])
                        n201 = Unbundle By Name(w260) -> ("Bay 4 Parameters.Resisdence time params"=w305:dbl[])
                        n202 = Unbundle By Name(w260) -> ("Bay 5 Parameters.Temperature Params"=w309:dbl[])
                        n203 = Unbundle By Name(w260) -> ("Bay 5 Parameters.Resisdence time params"=w304:dbl[])
                        n204 = Unbundle By Name(w260) -> ("Bay 1 Parameters.pump params 2"=w259:dbl[])
                        n205 = Unbundle By Name(w260) -> ("Bay 1 Parameters.pump params 1"=w308:dbl[])
                        n206 = Unbundle By Name(w260) -> ("Bay 3 Parameters.pump_num_ratio"=w288:dbl)
                        n207 = Unbundle By Name(w260) -> ("Bay 4 Parameters.pump_num_ratio"=w285:dbl)
                        n208 = Unbundle By Name(w260) -> ("Bay 5 Parameters.pump_num_ratio"=w282:dbl)
                        n209 = Unbundle By Name(w260) -> ("Bay 2 Parameters.pump_num_ratio"=w291:dbl)
                        n210 = Unbundle By Name(w260) -> ("Bay 4 Parameters.pump_at_ratio"=w287:bool)
                        n211 = Boolean To (0,1)(Boolean=w287) -> (0, 1=w286:i16)
                        n212 = Unbundle By Name(w260) -> ("Bay 3 Parameters.pump_at_ratio"=w290:bool)
                        n213 = Boolean To (0,1)(Boolean=w290) -> (0, 1=w289:i16)
                        n214 = Unbundle By Name(w260) -> ("Bay 5 Parameters.pump_at_ratio"=w284:bool)
                        n215 = Boolean To (0,1)(Boolean=w284) -> (0, 1=w283:i16)
                        n216 = Unbundle By Name(w260) -> ("Bay 2 Parameters.pump_at_ratio"=w293:bool)
                        n217 = Boolean To (0,1)(Boolean=w293) -> (0, 1=w292:i16)
                        n218 = script code="length_reactor1 = 188;%cm\nsystem_error = 0;\nlength_reactor2 = 99; %cm\nlength_bypass = 10;%cm\nnumPeaks = 1;\nstart_phase_time = 1;\nis_redo_exp = 0;\nFvalues = [];\nHPLC_Area = [];\ntube_diameters = [.01, .02, .03, .04];\nD1 = tube_diameters(tube_id(1) +1); D1 = D1*2.54;\nD2 = tube_diameters(tube_id(2) +1); D2 = D2*2.54;\nD3 = tube_diameters(tube_id(3) +1); D3 = D3*2.54;\nD4 = tube_diameters(tube_id(4) +1); D4 = D4*2.54;\nD5 = tube_diameters(tube_id(5) +1); D5 = D5*2.54;\nT1_span = [1 1]; T2_span = [1 1]; T3_span = [1 1]; T4_span = [1 1]; T5_span = [1 1];\n p1_span =  [1 1]; p2_span =  [1 1]; p3_span =  [1 1]; p4_span =  [1 1]; p5_span =  [1 1];  p6_span =  [1 1];\nOpt_params = [0 0 0 0 0 0 0 0 0 0 0];\nopt_ctr = 0;ncall = 100;\nrecord_data = true;\nT1_SP = 23; T2_SP = 23; T3_SP = 23; T4_SP = 23; T5_SP = 23;\nno_errors = 1;\nP1 = 0; P2 =0; P3 = 0; P4 = 0; P5 = 0; P6 = 0;\nis_first_set_of_exp = true;\nerror_message = 'System has no errors to report';\n%addpath(genpath('C:\\Users\\HPLC\\Dropbox (MIT)\\multistep_optimization'))\naddpath(genpath('C:\\Users\\HPLC\\Dropbox (MIT)\\MoD Files\\MATLAB'))\nallMSData = [];\nallHPLCData = [];\nallHPLCFile = [];\nCurrExp = 1;\nif Continue\n   load(matlabsavefile);\nelse\nx = []\n   IRSteadystate = 0;\n   ProductVec = [];\n   TwopointbaselineProductVec=[];\nend\nall_MSData = [];\n% ****************************************************************************************************\nif Bay1 == 1\n    %1.05m reactor\n     Vr1 = length_reactor1*D1^2/4*3.14159*1000;\n     if  Optimize_params(1)\n       % if choice is made to optimize temperature\n        if T1_params(2) < T1_params(3)\n             T1_span = [T1_params(2) ,  T1_params(3)];\n              Opt_params(1) = 1;\n         else\n            no_errors = 0;\n            error_message = 'Lower bound of temperature must be lower than upper bound';\n        end\n    else\n       %  if choice is made to not optimize temperature\n        T1_SP = T1_params(1);  \n    end\n\n    if Optimize_params(2)\n       % if user wants to optimize flowrates\n        if pump1_params(2) < pump1_params(3)\n             p1_span = [pump1_params(2) ,  pump1_params(3)];\n             p1_span = p1_span;\n             Opt_params(6) = 1; Opt_params(7) = 1;\n         else\n            no_errors = 0;\n            error_message = 'Lower bound of flowrate 1 must be lower than upper bound';\n        end\n         if pump2_params(2) < pump2_params(3)\n             p2_span = [pump2_params(2) ,  pump2_params(3)];\n             p2_span = p2_span;\n             Opt_params(6) = 1; Opt_params(7) = 1;\n         else\n            no_errors = 0;\n            error_message = 'Lower bound of flowrate 2 must be lower than upper bound';\n        end \n    else\n       if use_flowrate1\n            if P1_setrate < 0 || P2_setrate < 0\n               no_errors = 0;\n               error_message = 'Pump set flowrates can not be negative';\n            else\n               P1 = P1_setrate;\n               P2 = P1_setrate;\n            end\n       else\n            if pump1_params(1) > 0\n               P1 = pump1_params(1);\n            elseif not(isempty(pump1_chem))\n               no_errors = 0;\n               error_message = 'Bay1 Pump 1 setpoint must be greater than zero';\n            end\n             if pump2_params(1) > 0\n               P2 = pump2_params(1);\n            elseif not(isempty(pump2_chem))\n               no_errors = 0;\n               error_message = 'Bay1 Pump 2 setpoint must be greater than zero';\n            end\n       end\n    end\nelseif Bay1 == 0\n    % .1m bypass\n    Vr1 =length_bypass*D1^2/4*3.14159*1000;\n    if Optimize_params(1)\n          no_errors = 0;\n          error_message = 'Can not optimize temperature on bypass ';\n    end\n\n    if Optimize_params(2)\n       % if user wants to optimize residence time\n        if pump1_params(2) < pump1_params(3)\n             p1_span = [pump1_params(2) ,  pump1_params(3)];\n             p1_span = p1_span;\n             Opt_params(6) = 1; Opt_params(7) = 1;\n         else\n            no_errors = 0;\n            error_message = 'Lower bound of pump 1 must be lower than upper bound';\n        end\n       if pump2_params(2) < pump2_params(3)\n             p2_span = [pump2_params(2) ,  pump2_params(3)];\n             p2_span = p2_span;\n             Opt_params(6) = 1; Opt_params(7) = 1;\n         else\n            no_errors = 0;\n            error_message = 'Lower bound of pump 2 must be lower than upper bound';\n        end\n    else\n       if use_flowrate1\n            if P1_setrate < 0 || P2_setrate < 0\n               no_errors = 0;\n               error_message = 'Pump set flowrates can not be negative';\n            else\n               P1 = P1_setrate;\n               P2 = P2_setrate;\n            end\n       else\n            if pump1_params(1) > 0\n               P1 = pump1_params(1);\n            elseif not(isempty(pump1_chem))\n               no_errors = 0;\n               error_message = 'Bay 1 Pump 2 setpoint must be greater than zero';\n            end\n           if pump2_params(1) > 0\n               P2 = pump2_params(1);\n            elseif not(isempty(pump2_chem))\n               no_errors = 0;\n               error_message = 'Bay 1 Pump 2 setpoint must be greater than zero';\n            end\n       end\n    end\nelse\n    %separator\n    Vr1 = 1000;\n    if use_flowrate1\n        P1 = P1_setrate;\n        P2 = P2_setrate;\n    else \n        if not(isempty(pump1_chem))\n           P1 = 200;\n        end\n        if not(isempty(pump2_chem))\n           P2 = 200;\n        end\n    end\n    \nend\n\n% ****************************************************************************************************\n\n   if Bay2 == 1 \n   %1.05m reactor\n     Vr2 =length_reactor1*D2^2/4*3.14159*1000;\n     if  Optimize_params(3)\n       % if choice is made to optimize temperature\n        if T2_params(2) < T2_params(3)\n             T2_span = [T2_params(2) ,  T2_params(3)];\n             Opt_params(2) = 1;\n         else\n            no_errors = 0;\n            error_message = 'Lower bound of temperature must be lower than upper bound';\n        end\n    else\n       %  if choice is made to not optimize temperature\n        T2_SP = T2_params(1);  \n    end\n\n    if Optimize_params(4)\n       % if user wants to optimize residence time\n        if pump3_params(2) < pump3_params(3)\n             p3_span = [pump3_params(2) ,  pump3_params(3)];\n             p3_span = p3_span;\n             Opt_params(8) = 1;\n         else\n            no_errors = 0;\n            error_message = 'Lower bound of pump 3 must be lower than upper bound';\n        end\n    else\n       if use_flowrate2\n            if P3_setrate < 0\n               no_errors = 0;\n               error_message = 'Pump set flowrates can not be negative';\n            else\n               P3 = P3_setrate;\n            end\n       elseif Bay2_ratio\n            P3 = Bay2_pump_ratio*(P1); % changed from Bay2_pump_ratio*(P1+P2); \n       else\n            if pump3_params(1) > 0\n               P3 = pump3_params(1);\n            elseif not(isempty(pump3_chem))\n               no_errors = 0;\n               error_message = 'Bay 2 Pump 3 flowrate setpoint must be greater than zero';\n            end\n       end\n    end\nelseif Bay2 == 0\n    % .1m bypass\n    Vr2 =length_bypass*D2^2/4*3.14159*1000;\n    if Optimize_params(3)\n          no_errors = 0;\n          error_message = 'Can not optimize temperature on bypass ';\n    end\n\n    if Optimize_params(4)\n       % if user wants to optimize residence time\n        if pump3_params(2) < pump3_params(3)\n             p3_span = [pump3_params(2) ,  pump3_params(3)];\n             p3_span = p3_span;\n             Opt_params(8) = 1;\n         else\n            no_errors = 0;\n            error_message = 'Lower bound of resisdence time must be lower than upper bound';\n        end\n    else\n       if use_flowrate2\n            if P3_setrate < 0\n               no_errors = 0;\n               error_message = 'Pump set flowrates can not be negative';\n            else\n               P3 = P3_setrate;\n            end\n      elseif Bay2_ratio\n           P3 = Bay2_pump_ratio*(P1); % changed from Bay2_pump_ratio*(P1+P2); \n       else\n            if pump3_params(1) > 0\n               P3 = pump3_params(1);\n            elseif not(isempty(pump3_chem))\n               no_errors = 0;\n               error_message = 'Bay 2 Pump 3 setpoint must be greater than zero';\n            end\n       end\n    end\n   else\n    %separator\n    Vr2 = 1000;\n    if Optimize_params(4)\n       % if user wants to optimize residence time\n        if pump3_params(2) < pump3_params(3)\n             p3_span = [pump3_params(2) ,  pump3_params(3)];\n             p3_span = p3_span;\n             Opt_params(8) = 1;\n         else\n            no_errors = 0;\n            error_message = 'Lower bound of pump flowrate must be lower than upper bound';\n        end\n    else\n       if use_flowrate2\n           P3 = P3_setrate;\n       elseif Bay3_ratio\n           P3 = Bay2_pump_ratio*(P1); % changed from Bay2_pump_ratio*(P1+P2); \n       elseif not(isempty(pump3_chem))\n          P3 = 200;\n        end\n      end\n   end\n\n% ****************************************************************************************************\n\n  if Bay3 == 1 \n   %1.05m reactor\n     Vr3= length_reactor1*D3^2/4*3.14159*1000;\n     Vr3 = 1300;\n     if  Optimize_params(5)\n       % if choice is made to optimize temperature\n        if T3_params(2) < T3_params(3)\n             T3_span = [T3_params(2) ,  T3_params(3)];\n             Opt_params(3) = 1;\n         else\n            no_errors = 0;\n            error_message = 'Lower bound of temperature must be lower than upper bound';\n        end\n    else\n       %  if choice is made to not optimize temperature\n        T3_SP = T3_params(1);  \n    end\n\n    if Optimize_params(6)\n       % if user wants to optimize residence time\n        if pump4_params(2) < pump4_params(3)\n             p4_span = [pump4_params(2) ,  pump4_params(3)];\n             p4_span = p4_span;\n             Opt_params(9) = 1;\n         else\n            no_errors = 0;\n            error_message = 'Lower bound of pump 4 flowrate must be lower than upper bound';\n        end\n    else\n       if use_flowrate3\n            if P4_setrate < 0\n               no_errors = 0;\n               error_message = 'Pump set flowrates can not be negative';\n            else\n               P4 = P4_setrate;\n            end\n       elseif Bay3_ratio\n            P4= Bay3_pump_ratio*(P1+P2+P3);\n       else\n            if pump4_params(1) > 0\n               %Should a check be made whether or not tau1 > tau2\n                 P4 = pump4_params(1) ;\n            elseif not(isempty(pump4_chem))\n               no_errors = 0;\n               error_message = 'Bay 3 pump 4 setpoint must be greater than zero';\n            end\n       end\n    end\nelseif Bay3 == 0\n    % .1m bypass\n    Vr3 =length_bypass*D3^2/4*3.14159*1000;\n    if Optimize_params(5)\n          no_errors = 0;\n          error_message = 'Can not optimize temperature on bypass ';\n    end\n\n    if Optimize_params(6)\n       % if user wants to optimize residence time\n        if pump4_params(2) < pump4_params(3)\n             p4_span = [pump4_params(2) ,  pump4_params(3)];\n             p4_span = p4_span;\n             Opt_params(9) = 1;\n         else\n            no_errors = 0;\n            error_message = 'Lower bound of pump 4 setpoint must be lower than upper bound';\n        end\n    else\n       if use_flowrate3\n            if P4_setrate < 0\n               no_errors = 0;\n               error_message = 'Pump set flowrates can not be negative';\n            else\n               P4 = P4_setrate;\n            end\n       elseif Bay3_ratio\n            P4= Bay3_pump_ratio*(P1+P2+P3);\n       else\n            if pump4_params(1) > 0\n               P4 =pump4_params(1) ;\n            elseif not(isempty(pump4_chem))\n               no_errors = 0;\n               error_message = 'Bay 3 pump 4 setpoint must be greater than zero';\n            end\n       end\n    end\n   else\n    %separator\n      Vr3 = 1000;\n      if Optimize_params(6)\n       % if user wants to optimize residence time\n        if pump4_params(2) < pump4_params(3)\n             p4_span = [pump4_params(2) ,  pump4_params(3)];\n             p4_span = p4_span;\n             Opt_params(9) = 1;\n         else\n            no_errors = 0;\n            error_message = 'Lower bound of pump 4 flowrate must be lower than upper bound';\n        end\n     else\n        if use_flowrate3\n           P4 = P4_setrate;\n        elseif Bay3_ratio\n            P4= Bay3_pump_ratio*(P1+P2+P3);\n        elseif not(isempty(pump4_chem))\n          P4 = 200;\n        end\n      end\n   end\n\n% ****************************************************************************************************\n\n   if Bay4 == 1 \n   %1.05m reactor\n     Vr4 = length_reactor2*D4^2/4*3.14159*1000;\n     if  Optimize_params(7)\n       % if choice is made to optimize temperature\n        if T4_params(2) < T4_params(3)\n             T4_span = [T4_params(2) ,  T4_params(3)];\n              Opt_params(4) = 1;\n         else\n            no_errors = 0;\n            error_message = 'Lower bound of temperature must be lower than upper bound';\n        end\n    else\n       %  if choice is made to not optimize temperature\n        T4_SP = T4_params(1);  \n    end\n\n    if Optimize_params(8)\n       % if user wants to optimize residence time\n        if pump5_params(2) < pump5_params(3)\n             p5_span = [pump5_params(2) ,  pump5_params(3)];\n             p5_span = p5_span;\n            Opt_params(10) = 1;\n         else\n            no_errors = 0;\n            error_message = 'Lower bound of pump 5 flowrate must be lower than upper bound';\n        end\n    else\n       if use_flowrate4\n            if P5_setrate < 0\n               no_errors = 0;\n               error_message = 'Pump set flowrates can not be negative';\n            else\n               P5 = P5_setrate;\n            end\n       elseif Bay4_ratio\n            P5= Bay4_pump_ratio*(P1+P2+P3+P4);\n       else\n            if pump5_params(1) > 0\n               %Should a check be made whether or not tau4 > tau3\n                 P5 = pump5_params(1) ;\n            elseif not(isempty(pump5_chem))\n               no_errors = 0;\n               error_message = 'Bay 4 Pump 5 setpoint must be greater than zero';\n            end\n       end\n    end\nelseif Bay4 == 0\n    % .1m bypass\n    Vr4 =length_bypass*D4^2/4*3.14159*1000;\n    if Optimize_params(7)\n          no_errors = 0;\n          error_message = 'Can not optimize temperature on bypass ';\n    end\n\n    if Optimize_params(8)\n       % if user wants to optimize residence time\n        if pump5_params(2) < pump5_params(3)\n             p5_span = [pump5_params(2) ,  pump5_params(3)];\n             p5_span = p5_span;\n             Opt_params(10) = 1;\n         else\n            no_errors = 0;\n            error_message = 'Lower bound of resisdence time must be lower than upper bound';\n        end\n    else\n       if use_flowrate4\n            if P5_setrate < 0\n               no_errors = 0;\n               error_message = 'Pump set flowrates can not be negative';\n            else\n               P5 = P5_setrate;\n            end\n       elseif Bay4_ratio\n            P5= Bay4_pump_ratio*(P1+P2+P3+P4);\n       else\n            if pump5_params(1) > 0\n               P5 = pump5_params(1);\n            elseif not(isempty(pump5_chem))\n               no_errors = 0;\n               error_message = 'Bay 4 pump 5 setpoint must be greater than zero';\n            end\n       end\n    end\n   else\n    %separator\n      Vr4 = 1000;\n      if Optimize_params(8)\n       % if user wants to optimize residence time\n         if pump5_params(2) < pump5_params(3)\n             p5_span = [pump5_params(2) ,  pump5_params(3)];\n             p5_span = p5_span;\n             Opt_params(10) = 1;\n         else\n            no_errors = 0;\n            error_message = 'Lower bound of resisdence time must be lower than upper bound';\n         end\n       else\n           if use_flowrate4\n              P5 = P5_setrate;\n           elseif Bay4_ratio\n              P5= Bay4_pump_ratio*(P1+P2+P3+P4);\n           elseif not(isempty(pump5_chem))\n              P5 = 200;\n           end\n        end\n   end\n\n% ****************************************************************************************************\n\n  if Bay5 == 1 \n   %1.05m reactor\n     Vr5= length_reactor*D5^2/4*3.14159*1000;\n     if  Optimize_params(9)\n       % if choice is made to optimize temperature\n        if T5_params(2) < T5_params(3)\n             T5_span = [T5_params(2) ,  T5_params(3)];\n             Opt_params(5) = 1;\n         else\n            no_errors = 0;\n            error_message = 'Lower bound of temperature must be lower than upper bound';\n        end\n    else\n       %  if choice is made to not optimize temperature\n        T5_SP = T5_params(1);  \n    end\n\n    if Optimize_params(10)\n       % if user wants to optimize residence time\n        if pump6_params(2) < pump6_params(3)\n             p6_span = [pump6_params(2) ,  pump6_params(3)];\n             p6_span = p6_span;\n             Opt_params(11) = 1;\n         else\n            no_errors = 0;\n            error_message = 'Lower bound of pump 6 flowrate must be lower than upper bound';\n        end\n    else\n       if use_flowrate5\n            if P6_setrate < 0\n               no_errors = 0;\n               error_message = 'Pump set flowrates can not be negative';\n            else\n               P6 = P6_setrate;\n            end\n      elseif Bay5_ratio\n              P6= Bay5_pump_ratio*(P1+P2+P3+P4+P5);\n      else\n            if pump6_params(1) > 0\n               %Should a check be made whether or not tau1 > tau2\n                 P6 =pump6_params(1) ;\n            elseif not(isempty(pump6_chem))\n               no_errors = 0;\n               error_message = 'Bay 5 pump 6 setpoint must be greater than zero';\n            end\n       end\n    end\nelseif Bay5 == 0\n    % .1m bypass\n    Vr5 =length_bypass*D5^2/4*3.14159*1000;\n    if Optimize_params(9)\n          no_errors = 0;\n          error_message = 'Can not optimize temperature on bypass ';\n    end\n\n    if Optimize_params(10)\n       % if user wants to optimize residence time\n        if pump6_params(2) < pump6_params(3)\n             p6_span = [pump6_params(2) ,  pump6_params(3)];\n             p6_span = p6_span;\n             Opt_params(11) = 1;\n         else\n            no_errors = 0;\n            error_message = 'Lower bound of pump 6 must be lower than upper bound';\n        end\n    else\n       if use_flowrate5\n            if P6_setrate < 0\n               no_errors = 0;\n               error_message = 'Pump set flowrates can not be negative';\n            else\n               P6 = P6_setrate;\n            end\n      elseif Bay5_ratio\n              P6= Bay5_pump_ratio*(P1+P2+P3+P4+P5);\n       else\n            if pump6_params(1) > 0\n               P6 = pump6_params(1);\n            elseif not(isempty(pump6_chem))\n               no_errors = 0;\n               error_message = 'Bay 5 pump 6 setpoint must be greater than zero';\n            end\n       end\n    end\n   else\n    %separator\n      Vr5 = 1000;\n      if Optimize_params(10)\n       % if user wants to optimize residence time\n        if pump6_params(2) < pump6_params(3)\n             p6_span = [pump6_params(2) ,  pump6_params(3)];\n             p6_span = p6_span;\n             Opt_params(11) = 1;\n         else\n            no_errors = 0;\n            error_message = 'Lower bound of pump 6 must be lower than upper bound';\n        end\n      else\n         if use_flowrate5\n               P6 = P6_setrate;\n         elseif Bay5_ratio\n               P6= Bay5_pump_ratio*(P1+P2+P3+P4+P5);\n         elseif not(isempty(pump6_chem))\n              P6 = 200;\n         end\n      end\n   end\n\n% ****************************************************************************************************\n\n%Setup optimization\n\n   initialize_opt = 0;\n\n%*****************************************************************************************************\n% Setup excel and xml file writing\n\npath(path, pa);\nnumMSSig = 1;\n\n%Setup output excel file\n% Opening Excel file and inputing first peaks headers if needed\ntry\n  xlApp = actxGetRunningServer('Excel.Application');\ncatch ME\n  xlApp = actxserver('Excel.Application');\nend\n\nxlApp.DisplayAlerts = false; \nxlApp.Visible = false;\n\n%try\n   xlWorkbook = xlApp.workbooks.Open(xl_file, 0,false);\n   xlSheets = xlWorkbook.Sheets;\n   xlSheetNamesArray = cell(xlSheets.Count, 1);\n\n  for i = 1:xlSheets.Count\n     xlSheetNamesArray{i} = xlSheets.Item(i).Name;\n  end\n\n  [~, idx1] = ismember('Time_Series_Conditions', xlSheetNamesArray);\n  lastcol1 = xlcolumnletter(22);\n\n  [~, idx2] = ismember('MS Results', xlSheetNamesArray);\n  lastcol2 = xlcolumnletter(2);\n\n  [~, idx3] = ismember('System Setup', xlSheetNamesArray);\n  lastcol3 = xlcolumnletter(11);\n\n  [~, idx4] = ismember('HPLC Results', xlSheetNamesArray);\n  lastcol4 = xlcolumnletter(3);\n\n  [~, idx_ir_exp] = ismember('IR Results', xlSheetNamesArray);\n  IR_i= xlSheets.Item(idx_ir_exp).Range('A1').End('xlDown').Row ; \n  if IR_i == 1048576\n     IR_i = 2;\n  end\n \n  lastrow1 =  xlSheets.Item(idx1).Range('A1').End('xlDown').Row;\n  if lastrow1 == 1048576\n      lastrow1 = 2;\n  end\n\n  lastrow2 =  xlSheets.Item(idx2).Range('A1').End('xlDown').Row;\n  if lastrow2 == 1048576\n      lastrow2 = 2;\n  end\n\n   lastrow3= 2;\n\n    lastrow4=  xlSheets.Item(idx4).Range('A1').End('xlDown').Row;\n    if lastrow4 == 1048576\n       lastrow4 =2;\n    end\n\n%catch ME\n %   xlWorkbook = xlApp.Workbooks;\n %  xlWorkbook = invoke(xlWorkbook, 'Add');\n %   WS = xlWorkbook.Worksheets;\n %   row = num2str(1);\n %   temp_write = [Bay1, Bay2, Bay3, Bay4, Bay5, 1, Vr1, Vr2, Vr3, Vr4, Vr5];\n %   xlSheets.Item(idx3).Range(strcat('A',row,':',lastcol3,row)).Value2 =  temp_write;\n %   WS.Add([], WS.Item(WS.Count));\n %   WS.Item(WS.Count).Name = 'Time_Series_Conditions';\n %    WS.Add([], WS.Item(WS.Count));\n %    WS.Item(WS.Count).Name = 'MS Results';\n %   WS.Add([], WS.Item(WS.Count));\n %    WS.Item(WS.Count).Name = 'System Setup';\n %   WS.Add([], WS.Item(WS.Count));\n %    WS.Item(WS.Count).Name = 'HPLC Results';\n%end\n\nload('C:\\Users\\HPLC\\Dropbox (MIT)\\MoD Files\\MATLAB\\IR_Pks.mat');\n\ntemp_write = [Bay1, Bay2, Bay3, Bay4, Bay5, 1, Vr1, Vr2, Vr3, Vr4, Vr5];\nlastrowStr3 = num2str(lastrow3);\nxlSheets.Item(idx3).Range(strcat('A',lastrowStr3,':',lastcol3,lastrowStr3)).Value2 =  temp_write;\nlastrow3 = lastrow3 +1;\n\ntemp_write = {pump1_chem, pump2_chem, pump3_chem, pump4_chem, pump5_chem, pump6_chem};\nlastrowStr3 = num2str(6);\nxlSheets.Item(idx3).Range(strcat('B',lastrowStr3,':','G',lastrowStr3)).Value2 =  temp_write;\n\nlastrowStr3 = num2str(8);\nxlSheets.Item(idx3).Range(strcat('B',lastrowStr3,':','G',lastrowStr3)).Value2 = Pump_concen;\n\n\n\n%***************************************************************************************************\n\nredo = false;\nncall = ncall_in;"("Bay1"=w362, "Bay2"=w361, "Bay3"=w360, "Bay4"=w359, "Bay5"=w358, "tube_id"=w357, "use_flowrate1"=w344, "P1_setrate"=w356, "P2_setrate"=w355, "P3_setrate"=w354, "P4_setrate"=w353, "P5_setrate"=w352, "P6_setrate"=w351, "use_flowrate2"=w294, "use_flowrate3"=w341, "use_flowrate4"=w340, "use_flowrate5"=w337, "Optimize_params"=w316, "T1_params"=w313, "T2_params"=w312, "T3_params"=w311, "T4_params"=w310, "T5_params"=w309, "pump1_params"=w308, "pump3_params"=w307, "pump4_params"=w306, "pump5_params"=w305, "pump6_params"=w304, "P1_P2_ratio"=w301, "xml_file"=w300, "xl_file"=w299, "pa"=w298, "Continue"=w296, "matlabsavefile"=w295, "Bay2_ratio"=w292, "Bay2_pump_ratio"=w291, "Bay3_ratio"=w289, "Bay3_pump_ratio"=w288, "Bay4_ratio"=w286, "Bay4_pump_ratio"=w285, "Bay5_ratio"=w283, "Bay5_pump_ratio"=w282, "pump1_chem"=w274, "pump6_chem"=w273, "pump5_chem"=w272, "pump4_chem"=w271, "pump3_chem"=w270, "pump2_chem"=w269, "Pump_concen"=w262, "ncall_in"=w261, "pump2_params"=w259) -> ("Vr1"=w350:dbl, "Vr2"=w349:dbl, "Vr3"=w348:dbl, "Vr4"=w347:dbl, "Vr5"=w346:dbl, "no_errors"=w315:dbl, "error_message"=w314:string)  [unwired: 1 in, 1 out]
                        n219 = Not Equal To 0?(x=w315) -> (x != 0?=w302:bool)
                        n220 = Not(x=w302) -> (.not. x?=w303:bool)
                        n221 = case shown="True" w303 {
                          tunnel: w314 -> [_ w363]
                          frame False {
                          }
                          frame True {
                            n222 = One Button Dialog(message=w363) -> ()  [unwired: 1 in, 1 out]
                          }
                        }
                      }
                    }
                    n223 = local read "Stop"() -> (w234:bool)
                    n224 = Or(x=w226, y=w234) -> (x .or. y?=w235:bool)
                    n225 = Wait (ms)(milliseconds to wait=u32 500) -> ()  [unwired: 1 out]
                  }
                  n226 = local write "Volume (ul) 1"(w220) -> ()
                  n227 = local write "Volume (ul) 2"(w219) -> ()
                  n228 = local write "Volume (ul) 3"(w218) -> ()
                  n229 = local write "Volume (ul) 4"(w217) -> ()
                  n230 = local write "Volume (ul) 5"(w216) -> ()
                }
                frame #2 {
                  n231 = local write "Setup Confirm 2"(w364) -> ()
                }
              }
            }
          }
        }
        frame #2 {
          # "Run Initial diagnostics"
        }
        frame #3 {
          # "Run System"
          n232 = while {
            stop <- w954 stop-if-true
            n233 = local read "Debug_run_button"() -> (w950:bool)
            n234 = Not(x=w950) -> (.not. x?=w952:bool)
            n235 = local read "Temperature Control 1"() -> (w949:bool)
            n236 = And(x=w952, y=w949) -> (x .and. y?=w951:bool)
            n237 = case shown="True" w951 {
              frame False {
                n238 = local write "Temp SS? 1"(TRUE ("Temp SS? 1")) -> ()
              }
              frame True {
                # "Bay 1 Temperature Controller"
                n239 = local read "Temperature SP 1"() -> (w956:dbl)
                n240 = local read "Temperature 1"() -> (w960:dbl)
                n241 = local read "SSR Duration 1"() -> (w975:dbl)
                n242 = call-poly <vilib>:"PID Online Autotuning.vi"("setpoint"=w956, "manipulated variable"=w975, "autotuning parameters"=T8 {"type of controller"=enum."PID", "relay cycles"=3, "relay amplitude"=1.0, "control specifications"=enum."Normal", "PV noise level"=0.1} ("Autotuning Parameters R1"), "process variable"=w960, "PID gains in"=T7 {"Proportional gain Kc"=0.38538, "Integral time Ti (sec)"=0.524375, "Derivative time Ti (sec)"=0.12585} ("PID gains 2")) -> ("setpoint out"=w981:dbl, "process variable out"=w980:dbl, "PID gains out"=w977:T9)  [unwired: 6 in, 2 out]
                n243 = call <vilib>:"PID Autotuning (Temperature).vi"("desired temperature"=w981, "measured temperature"=w980, "plant parameters in"=w977, "output range"=cluster{"output high":dbl, "output low":dbl} {"output high"=3.0, "output low"=-1.0} ("Output range")) -> ("output"=w973:dbl)  [unwired: 12 in, 3 out]
                n244 = local write "SSR Duration 1"(w973) -> ()
                n245 = Subtract(x=w956, y=w960) -> (x-y=w967:dbl)
                n246 = Absolute Value(x=w967) -> (abs(x)=w970:dbl)
                n247 = Multiply(x=1000.0, y=w973) -> (x*y=w971:dbl)
                n248 = Greater Than 0?(x=w971) -> (x > 0?=w965:bool)
                n249 = Less Or Equal?(x=w970, y=1.2) -> (x <= y?=w968:bool)
                n250 = Greater?(x=w956, y=w960) -> (0:w966:bool)
                n251 = And(x=w965, y=w966) -> (x .and. y?=w963:bool)
                n252 = local write "Temp SS? 1"(w968) -> ()
                n253 = Subtract(x=w960, y=10.0) -> (x-y=w961:dbl)
                n254 = Less?(x=w961, y=w956) -> (x < y?=w964:bool)
                n255 = And(x=w964, y=w963) -> (x .and. y?=w962:bool)
                n256 = case shown="False" w962 {
                  tunnel: 2 -> [_ _]
                  tunnel: w971 -> [w985 _]
                  tunnel: [0.0 w988] -> w958
                  tunnel: w956 -> [_ w987]
                  frame False {
                    (unwired) errorcluster {"status"=FALSE, "code"=0, "source"=""} ("error out")
                    n257 = Absolute Value(x=w985) -> (abs(x)=w986:dbl)
                    n258 = Wait (ms)(milliseconds to wait=w986) -> ()  [unwired: 1 out]
                  }
                  frame True {
                    n259 = script code="tempdiff1= SP1 - T1;\nif tempdiff1 > 10\n  if slope1 < .01\n     temp_check1 = temp_check1 + 1;\n  else\n      temp_check1 =0;\n  end\nend\n\nif temp_check1 > 9\n  temp_error1 = 1\nend"("SP1"=w987) -> ("temp_error1"=w988:dbl)  [unwired: 1 in, 1 out]
                  }
                }
                n260 = Not Equal To 0?(x=w958) -> (x != 0?=w957:bool)
                n261 = case shown="True" w957 {
                  frame False {
                  }
                  frame True {
                    n262 = local write "Error Message"("Bay 1 Temperature Heating Error") -> ()
                  }
                }
                n263 = case shown="True" w957 {
                  tunnel: w957 -> [_ w983]
                  frame False {
                  }
                  frame True {
                    n264 = local write "Stop"(w983) -> ()
                  }
                }
              }
            }
            n265 = Wait (ms)(milliseconds to wait=u32 400) -> ()  [unwired: 1 out]
            n266 = local read "Stop"() -> (w954:bool)
          }
          n267 = local read "Bay Parameters"() -> (w368:T3)
          n268 = while {
            stop <- w914 stop-if-true
            n269 = local read "Debug_run_button"() -> (w910:bool)
            n270 = Not(x=w910) -> (.not. x?=w912:bool)
            n271 = local read "Temperature Control 2"() -> (w909:bool)
            n272 = And(x=w912, y=w909) -> (x .and. y?=w911:bool)
            n273 = case shown="True" w911 {
              frame False {
                n274 = local write "Temp SS? 2"(TRUE ("Temp SS? 2")) -> ()
              }
              frame True {
                # "Bay 2 Temperature Controller"
                n275 = local read "Temperature SP 2"() -> (w917:dbl)
                n276 = local read "Temperature 2"() -> (w920:dbl)
                n277 = local read "SSR Duration 2"() -> (w938:dbl)
                n278 = call-poly <vilib>:"PID Online Autotuning.vi"("setpoint"=w917, "manipulated variable"=w938, "autotuning parameters"=T8 {"type of controller"=enum."PID", "relay cycles"=3, "relay amplitude"=1.0, "control specifications"=enum."Normal", "PV noise level"=0.1} ("Autotuning Parameters R1"), "process variable"=w920, "PID gains in"=T7 {"Proportional gain Kc"=0.38538, "Integral time Ti (sec)"=0.524375, "Derivative time Ti (sec)"=0.12585} ("PID gains 2")) -> ("setpoint out"=w936:dbl, "process variable out"=w935:dbl, "PID gains out"=w941:T9)  [unwired: 6 in, 2 out]
                n279 = call <vilib>:"PID Autotuning (Temperature).vi"("desired temperature"=w936, "measured temperature"=w935, "plant parameters in"=w941, "output range"=cluster{"output high":dbl, "output low":dbl} {"output high"=3.0, "output low"=-1.0} ("Output range")) -> ("output"=w931:dbl)  [unwired: 12 in, 3 out]
                n280 = local write "SSR Duration 2"(w931) -> ()
                n281 = Greater?(x=w917, y=w920) -> (0:w926:bool)
                n282 = Multiply(x=1000.0, y=w931) -> (x*y=w933:dbl)
                n283 = Greater Than 0?(x=w933) -> (x > 0?=w925:bool)
                n284 = And(x=w925, y=w926) -> (x .and. y?=w923:bool)
                n285 = Subtract(x=w917, y=w920) -> (x-y=w928:dbl)
                n286 = Absolute Value(x=w928) -> (abs(x)=w930:dbl)
                n287 = Subtract(x=w920, y=10.0) -> (x-y=w922:dbl)
                n288 = Less Or Equal?(x=w930, y=1.2) -> (x <= y?=w927:bool)
                n289 = local write "Temp SS? 2"(w927) -> ()
                n290 = Less?(x=w922, y=w917) -> (x < y?=w924:bool)
                n291 = And(x=w924, y=w923) -> (x .and. y?=w919:bool)
                n292 = case shown="False" w919 {
                  tunnel: 3 -> [_ _]
                  tunnel: w933 -> [w945 _]
                  tunnel: [0.0 w948] -> w918
                  tunnel: w917 -> [_ w947]
                  frame False {
                    (unwired) errorcluster {"status"=FALSE, "code"=0, "source"=""} ("error out")
                    n293 = Absolute Value(x=w945) -> (abs(x)=w946:dbl)
                    n294 = Wait (ms)(milliseconds to wait=w946) -> ()  [unwired: 1 out]
                  }
                  frame True {
                    n295 = script code="tempdiff2= SP2 - T2;\nif tempdiff2 > 10\n  if slope2 < .01\n     temp_check2 = temp_check2 + 1;\n  else\n      temp_check2 =0;\n  end\nend\n\nif temp_check2 > 9\n  temp_error2 = 1\nend"("SP2"=w947) -> ("temp_error2"=w948:dbl)  [unwired: 1 in, 1 out]
                  }
                }
                n296 = Not Equal To 0?(x=w918) -> (x != 0?=w916:bool)
                n297 = case shown="True" w916 {
                  frame False {
                  }
                  frame True {
                    n298 = local write "Error Message"("Bay 2 Temperature Heating Error") -> ()
                  }
                }
                n299 = case shown="True" w916 {
                  tunnel: w916 -> [_ w943]
                  frame False {
                  }
                  frame True {
                    n300 = local write "Stop"(w943) -> ()
                  }
                }
              }
            }
            n301 = local read "Stop"() -> (w914:bool)
            n302 = Wait (ms)(milliseconds to wait=u32 400) -> ()  [unwired: 1 out]
          }
          n303 = local read "Stop"() -> (w365:bool)
          n304 = Not(x=w365) -> (.not. x?=w367:bool)
          n305 = case shown="True" w367 {
            tunnel: w368 -> [_ w372]
            tunnel: w366 -> [_ w371]
            frame False {
            }
            frame True {
              n306 = while {
                tunnel: w372 -> [w384]
                tunnel: w371 -> [w376]
                i -> [w383]
                stop <- w377 stop-if-true
                n307 = local read "Debug_run_button"() -> (w386:bool)
                n308 = Wait (ms)(milliseconds to wait=u32 1000) -> ()  [unwired: 1 out]
                n309 = Increment(x=w383) -> (x+1=w373:i32)
                n310 = case shown="False" w386 {
                  tunnel: w383 -> [_ w786]
                  tunnel: w384 -> [_ _]
                  tunnel: [w390 w788] -> w374
                  tunnel: [w391 0.0] -> w379
                  tunnel: w376 -> [w389 _]
                  frame False {
                    n311 = flat-sequence {
                      tunnel: w389 -> [w393]
                      tunnel: [w393] -> w388
                      tunnel: [w402] -> w391
                      tunnel: [200.0] -> w390
                      tunnel: w388 -> [w400]
                      frame #0 {
                        n312 = local write "stop_xl_write"(FALSE ("stop_xl_write")) -> ()
                      }
                      frame #1 {
                        # "Increase flowrate of dilution stream"
                        # "Wait mixed stream reaches SL"
                        # "SNOBFIT"
                        # "Optimize"
                        # "Run Experimental Conditions"
                        # "Optimize/Synthesize"
                        n313 = script code="if not(system_error)\n\nif not(redo)\n    % snobfit\n    snobfit_labview_driver;\n\n    if opt_ctr == 2\n      new_x = x(req_ctr,:);\n      x_ind = 1;\n      \n      if Opt_params(1)\n         T1_SP = new_x(x_ind ); %'C\n         params_1(1) = new_x(x_ind);\n         x_ind  = x_ind  + 1;\n      end\n     if Opt_params(2)\n       T2_SP = new_x(x_ind ); %'C\n        params_1(3) = new_x(x_ind);\n       x_ind  = x_ind  + 1;\n     end\n     if Opt_params(3)\n       T3_SP = new_x(x_ind ); %'C\n       x_ind  = x_ind  + 1;\n    end\n     if Opt_params(4)\n       T4_SP = new_x(x_ind ); %'C\n       x_ind  = x_ind  + 1;\n    end\n     if Opt_params(5)\n       T5_SP = new_x(x_ind ); %'C\n       x_ind  = x_ind  + 1;\n    end\n    if Opt_params(6)\n        tau1 = Vr1/(new_x( x_ind) +new_x( x_ind+1) );\n        %new_x( x_ind) = tau1*60;\n        params_1(2) = new_x(x_ind);\n        P2 =new_x( x_ind+1); %ul/min\n        P1=new_x( x_ind); %ul/min\n        x_ind  = x_ind  + 2;\n    end\n     if Opt_params(8)\n        tau2= Vr2/(new_x( x_ind)+P1+P2);\n        %new_x( x_ind) = tau2*60;\n        params_1(4) = new_x(x_ind);\n        P3=new_x( x_ind); %ul/minP2 = Vr4/(tau4)*60/2;\n        x_ind  = x_ind  + 1;\n      % P2 = Vr4/(tau4)*60/2;\n     elseif Bay2_ratio && not(use_flowrate2)\n        P3= Bay2_pump_ratio*(P1+P2); %chnaged from  P3= Bay2_pump_ratio*(P1 + P2);\n      end\n    if Opt_params(9)\n      tau3 =Vr3/(new_x( x_ind)+P1+P2+P3);\n      P4=new_x( x_ind); %ul/min\n      P3= Bay2_pump_ratio*(P4); \n      x_ind  = x_ind  + 1;\n    elseif Bay3_ratio && not(use_flowrate3)\n        P4= Bay3_pump_ratio*(P1+P2 +P3);\n    end\n    if Opt_params(10)\n      tau4 = Vr4/(new_x( x_ind)+P1+P2+P3+P4);\n      P5=new_x( x_ind) ; %ul/min\n       x_ind  = x_ind  + 1;\n    elseif Bay4_ratio && not(use_flowrate4)\n        P5= Bay4_pump_ratio*(P1+P2 +P3 +P4);\n    end\n    if Opt_params(11)\n      tau5 = Vr5/(new_x( x_ind)+P1+P2+P3+P4+P5);\n      %new_x( x_ind) = tau5*60;\n      P6=new_x( x_ind) ; %ul/min\n      x_ind  = x_ind  + 1;\n    elseif Bay5_ratio && not(use_flowrate5)\n        P6= Bay5_pump_ratio*(P1+P2 +P3 +P4 +P4 +P5);\n    end\n    %---------  \n end\n\n   P1=P1*2; P2 =P2*2; P3=P3*2; P4=P4*2; P5=P5*2; P6=P6*2;\n   Conditions_Array = [P1 P2 P3 P4 P5 P6 T1_SP T2_SP T3_SP T4_SP T5_SP];\n   if opt_ctr == 2\n        opt_ctr = 1;\n   else\n       opt_ctr = 2\n   end\nelse\n   opt_ctr =1;\n   redo = false;\n   is_redo_exp = 1;\n   if req_ctr ~= req_tot\n       req_ctr = req_ctr - 1;\n   end\n   CurrExp = CurrExp - 1;\n   ncall0 = ncall0 - 1;\n end\n\nend\n\nP_tot = P1 + P2 + P3 + P4 + P5 + P6 ;"() -> ("Conditions_Array"=w399:dbl[], "opt_ctr"=w405:dbl, "P_tot"=→"P_tot":dbl)  [unwired: 1 in, 1 out]
                        n314 = Not Equal To 0?(x=0.0) -> (x != 0?=w396:bool)
                        n315 = local write "Is current Exp a Redo?"(w396) -> ()
                        n316 = Not Equal To 0?(x=0.0) -> (x != 0?=w397:bool)
                        n317 = local write "Will Redo Next Exp?"(w397) -> ()
                        n318 = local read "COMM Port :: Milligat Pumps"() -> (w406:refnum<visa-resource-name>)
                        n319 = Equal?(x=w405, y=1.0) -> (x = y?=w403:bool)
                        n320 = flat-sequence {
                          tunnel: w399 -> [w741]
                          frame #0 {
                            # "Start recording data"
                            n321 = Index Array(array=w741, index=5) -> (element=w758:dbl)
                            n322 = Index Array(array=w741, index=0) -> (element=w750:dbl)
                            n323 = Index Array(array=w741, index=1) -> (element=w751:dbl)
                            n324 = Index Array(array=w741, index=2) -> (element=w756:dbl)
                            n325 = Index Array(array=w741, index=3) -> (element=w755:dbl)
                            n326 = Index Array(array=w741, index=4) -> (element=w757:dbl)
                            n327 = local read "Volume (ul) 3"() -> (w728:dbl)
                            n328 = local read "Volume (ul) 5"() -> (w726:dbl)
                            n329 = local read "Volume (ul) 4"() -> (w727:dbl)
                            n330 = local read "Volume (ul) 2"() -> (w729:dbl)
                            n331 = local read "Volume (ul) 1"() -> (w730:dbl)
                            n332 = Add(x=w750, y=w751) -> (x+y=w739:dbl)
                            n333 = Add(x=w739, y=w756) -> (x+y=w737:dbl)
                            n334 = Add(x=w737, y=w755) -> (x+y=w735:dbl)
                            n335 = Add(x=w735, y=w757) -> (x+y=w732:dbl)
                            n336 = Add(x=w732, y=w758) -> (x+y=w734:dbl)
                            n337 = local write "Pump setpoint(ul/min) 2"(w751) -> ()
                            n338 = local write "Pump setpoint(ul/min) 4"(w756) -> ()
                            n339 = local write "Pump setpoint(ul/min) 5"(w757) -> ()
                            n340 = Not Equal To 0?(x=w739) -> (x != 0?=w740:bool)
                            n341 = local write "Pump setpoint(ul/min) 3"(w755) -> ()
                            n342 = local write "Pump setpoint(ul/min) 6"(w758) -> ()
                            n343 = local write "Pump setpoint(ul/min) 1"(w750) -> ()
                            n344 = Not Equal To 0?(x=w734) -> (x != 0?=w731:bool)
                            n345 = Not Equal To 0?(x=w735) -> (x != 0?=w736:bool)
                            n346 = Not Equal To 0?(x=w732) -> (x != 0?=w733:bool)
                            n347 = Not Equal To 0?(x=w737) -> (x != 0?=w738:bool)
                            n348 = case shown="False" w738 {
                              tunnel: w737 -> [_ w774]
                              tunnel: [0.0 w773] -> w749
                              tunnel: w729 -> [_ w772]
                              frame False {
                              }
                              frame True {
                                n349 = Divide(x=w772, y=w774) -> (x/y=w773:dbl)
                              }
                            }
                            n350 = case shown="True" w731 {
                              tunnel: w734 -> [_ w766]
                              tunnel: [0.0 w765] -> w754
                              tunnel: w726 -> [_ w764]
                              frame False {
                              }
                              frame True {
                                n351 = Divide(x=w764, y=w766) -> (x/y=w765:dbl)
                              }
                            }
                            n352 = case shown="True" w736 {
                              tunnel: [0.0 w770] -> w752
                              tunnel: w735 -> [_ w769]
                              tunnel: w728 -> [_ w768]
                              frame False {
                              }
                              frame True {
                                n353 = Divide(x=w768, y=w769) -> (x/y=w770:dbl)
                              }
                            }
                            n354 = case shown="True" w740 {
                              tunnel: w739 -> [_ w780]
                              tunnel: [0.0 w777] -> w748
                              tunnel: w730 -> [_ w779]
                              frame False {
                              }
                              frame True {
                                n355 = Divide(x=w779, y=w780) -> (x/y=w778:dbl)
                                n356 = Multiply(x=w778, y=0.0) -> (x*y=w777:dbl)
                              }
                            }
                            n357 = case shown="True" w733 {
                              tunnel: w732 -> [_ w762]
                              tunnel: [0.0 w761] -> w753
                              tunnel: w727 -> [_ w760]
                              frame False {
                              }
                              frame True {
                                n358 = Divide(x=w760, y=w762) -> (x/y=w761:dbl)
                              }
                            }
                            n359 = local write "tau 2"(w749) -> ()
                            n360 = local write "tau 3"(w752) -> ()
                            n361 = local write "tau 4"(w753) -> ()
                            n362 = local write "tau 5"(w754) -> ()
                            n363 = local write "tau 1"(w748) -> ()
                          }
                        }
                        n364 = flat-sequence {
                          tunnel: w406 -> [w416]
                          tunnel: w399 -> [w415]
                          tunnel: w403 -> [w414]
                          tunnel: [w414] -> w412
                          tunnel: w400 -> [w413]
                          tunnel: w412 -> [w510]
                          tunnel: [w510] -> w411
                          tunnel: w411 -> [w530]
                          tunnel: [w528] -> w410
                          tunnel: w399 -> [w563]
                          tunnel: w410 -> [w562]
                          tunnel: [w680] -> w409
                          tunnel: w409 -> [w683]
                          tunnel: [w683] -> w408
                          tunnel: w408 -> [w691]
                          tunnel: [w691] -> w407
                          tunnel: [w725] -> w402
                          tunnel: w407 -> [w725]
                          frame #0 {
                            # "Setup pump flowrates and temperature setpoints"
                            n365 = stacked-sequence {
                              tunnel: w416 -> [w433 _ _ _ _]
                              tunnel: w416 -> [_ w455 _ _ _]
                              tunnel: w416 -> [_ _ w471 _ _]
                              tunnel: w416 -> [_ _ _ w487 _]
                              tunnel: w416 -> [_ _ _ _ w505]
                              tunnel: w415 -> [w430 w453 w469 w485 w500]
                              tunnel: w414 -> [w419 w445 w461 w477 w493]
                              tunnel: w413 -> [w417 _ _ _ _]
                              frame #0 {
                                # "Bay 1"
                                n366 = local read "Syringe_pump?"() -> (w418:bool)
                                n367 = Index Array(array=w430, index=0) -> (element=w428:dbl)
                                n368 = local read "Bay 1"() -> (w435:u16)
                                n369 = Index Array(array=w430, index=1) -> (element=w427:dbl)
                                n370 = Index Array(array=w430, index=6) -> (element=w426:dbl)
                                n371 = script code="MATLAB script"("P1"=w428, "P2"=w427, "T1_SP"=w426) -> ()  [unwired: 1 in, 1 out]
                                n372 = Greater Than 0?(x=w428) -> (x > 0?=w425:bool)
                                n373 = And(x=w425, y=w419) -> (x .and. y?=w424:bool)
                                n374 = Greater Than 0?(x=w427) -> (x > 0?=w423:bool)
                                n375 = Equal?(x=w435, y=u16 1) -> (x = y?=w421:bool)
                                n376 = And(x=w423, y=w419) -> (x .and. y?=w422:bool)
                                n377 = And(x=w421, y=w419) -> (x .and. y?=w420:bool)
                                n378 = case shown="False" w418 {
                                tunnel: w433 -> [w438 _]
                                tunnel: w427 -> [w437 w440]
                                tunnel: w422 -> [w436 w441]
                                tunnel: w417 -> [_ w439]
                                frame False {
                                n379 = case shown="False" w436 {
                                tunnel: w438 -> [_ _]
                                tunnel: w437 -> [_ _]
                                frame False {
                                }
                                frame True {
                                }
                                }
                                }
                                frame True {
                                n380 = case shown="True" w441 {
                                tunnel: w440 -> [_ _]
                                tunnel: w439 -> [_ _]
                                frame False {
                                }
                                frame True {
                                }
                                }
                                }
                                }
                                n381 = case shown="False" w424 {
                                tunnel: w433 -> [_ _]
                                tunnel: w428 -> [_ _]
                                frame False {
                                }
                                frame True {
                                # "switched j and g"
                                }
                                }
                                n382 = case shown="True" w420 {
                                tunnel: w426 -> [_ w444]
                                frame False {
                                n383 = local write "Temperature Control 1"(FALSE) -> ()
                                }
                                frame True {
                                n384 = local write "Temperature SP 1"(w444) -> ()
                                n385 = local write "Temperature Control 1"(TRUE ("Temperature Control 1")) -> ()
                                }
                                }
                              }
                              frame #1 {
                                # "Bay 2"
                                n386 = Index Array(array=w453, index=2) -> (element=w450:dbl)
                                n387 = Index Array(array=w453, index=7) -> (element=w451:dbl)
                                n388 = script code="MATLAB script"("T2_SP"=w451, "P3"=w450) -> ()  [unwired: 1 in, 1 out]
                                n389 = local read "Bay 2"() -> (w456:u16)
                                n390 = Equal?(x=w456, y=u16 1) -> (x = y?=w449:bool)
                                n391 = Greater Than 0?(x=w450) -> (x > 0?=w447:bool)
                                n392 = And(x=w449, y=w445) -> (x .and. y?=w448:bool)
                                n393 = And(x=w447, y=w445) -> (x .and. y?=w446:bool)
                                n394 = case shown="True" w448 {
                                tunnel: w451 -> [_ w459]
                                frame False {
                                n395 = local write "Temperature Control 2"(FALSE) -> ()
                                }
                                frame True {
                                n396 = local write "Temperature Control 2"(TRUE ("Temperature Control 2")) -> ()
                                n397 = local write "Temperature SP 2"(w459) -> ()
                                }
                                }
                                n398 = case shown="False" w446 {
                                tunnel: w450 -> [_ _]
                                tunnel: w455 -> [_ _]
                                frame False {
                                }
                                frame True {
                                }
                                }
                              }
                              frame #2 {
                                # "Bay 3"
                                n399 = Index Array(array=w469, index=3) -> (element=w466:dbl)
                                n400 = local read "Bay 3"() -> (w473:u16)
                                n401 = Not Equal To 0?(x=w466) -> (x != 0?=w465:bool)
                                n402 = Index Array(array=w469, index=8) -> (element=w467:dbl)
                                n403 = script code="MATLAB script"("T3_SP"=w467, "P4"=w466) -> ()  [unwired: 1 in, 1 out]
                                n404 = Equal?(x=w473, y=u16 1) -> (x = y?=w463:bool)
                                n405 = And(x=w463, y=w461) -> (x .and. y?=w462:bool)
                                n406 = And(x=w465, y=w461) -> (x .and. y?=w464:bool)
                                n407 = case shown="True" w462 {
                                tunnel: w467 -> [_ w475]
                                frame False {
                                n408 = local write "Temperature Control 3"(FALSE) -> ()
                                }
                                frame True {
                                n409 = local write "Temperature Control 3"(TRUE ("Temperature Control 3")) -> ()
                                n410 = local write "Temperature SP 3"(w475) -> ()
                                }
                                }
                                n411 = case shown="True" w464 {
                                tunnel: w466 -> [_ _]
                                tunnel: w471 -> [_ _]
                                frame False {
                                }
                                frame True {
                                }
                                }
                              }
                              frame #3 {
                                # "Bay 4"
                                n412 = Index Array(array=w485, index=9) -> (element=w482:dbl)
                                n413 = Index Array(array=w485, index=4) -> (element=w483:dbl)
                                n414 = script code="MATLAB script"("P5"=w483, "T4_SP"=w482) -> ()  [unwired: 1 in, 1 out]
                                n415 = Not Equal To 0?(x=w483) -> (x != 0?=w481:bool)
                                n416 = local read "Bay 4"() -> (w488:u16)
                                n417 = Equal?(x=w488, y=1) -> (x = y?=w478:bool)
                                n418 = And(x=w481, y=w477) -> (x .and. y?=w480:bool)
                                n419 = And(x=w478, y=w477) -> (x .and. y?=w479:bool)
                                n420 = case shown="False" w480 {
                                tunnel: w487 -> [_ _]
                                tunnel: w483 -> [_ _]
                                frame False {
                                }
                                frame True {
                                }
                                }
                                n421 = case shown="True" w479 {
                                tunnel: w482 -> [_ w491]
                                frame False {
                                n422 = local write "Temperature Control 4"(FALSE ("Temperature Control 4")) -> ()
                                }
                                frame True {
                                n423 = local write "Temperature SP 4"(w491) -> ()
                                n424 = local write "Temperature Control 4"(TRUE ("Temperature Control 5")) -> ()
                                }
                                }
                              }
                              frame #4 {
                                # "Bay 5"
                                n425 = Index Array(array=w500, index=5) -> (element=w498:dbl)
                                n426 = Index Array(array=w500, index=4) -> (element=w499:dbl)
                                n427 = script code="MATLAB script"("T5_SP"=w499, "P6"=w498) -> ()  [unwired: 1 in, 1 out]
                                n428 = Not Equal To 0?(x=w498) -> (x != 0?=w495:bool)
                                n429 = And(x=w495, y=w493) -> (x .and. y?=w494:bool)
                                n430 = local read "Bay 5"() -> (w504:u16)
                                n431 = Equal?(x=w504, y=u16 1) -> (x = y?=w496:bool)
                                n432 = And(x=w496, y=w493) -> (x .and. y?=w497:bool)
                                n433 = case shown="True" w497 {
                                tunnel: w499 -> [_ w507]
                                frame False {
                                n434 = local write "Temperature Control 5"(FALSE ("Temperature Control 5")) -> ()
                                }
                                frame True {
                                n435 = local write "Temperature SP 5"(w507) -> ()
                                n436 = local write "Temperature Control 5"(TRUE ("Temperature Control 5")) -> ()
                                }
                                }
                                n437 = case shown="True" w494 {
                                tunnel: w505 -> [_ _]
                                tunnel: w498 -> [_ _]
                                frame False {
                                }
                                frame True {
                                }
                                }
                              }
                            }
                          }
                          frame #1 {
                            # "Wait till Steady State temperature readings on all bays"
                            n438 = while {
                              tunnel: w510 -> [w511]
                              stop <- w512 stop-if-true
                              n439 = flat-sequence {
                                tunnel: [w515] -> w512
                                tunnel: w511 -> [w514]
                                frame #0 {
                                n440 = Wait (ms)(milliseconds to wait=u32 1500) -> ()  [unwired: 1 out]
                                }
                                frame #1 {
                                n441 = local read "Temp SS? 2"() -> (w518:bool)
                                n442 = local read "Temp SS? 3"() -> (w519:bool)
                                n443 = local read "Temp SS? 4"() -> (w520:bool)
                                n444 = local read "Temp SS? 5"() -> (w521:bool)
                                n445 = local read "Temp SS? 1"() -> (w517:bool)
                                n446 = Not(x=w514) -> (.not. x?=w527:bool)
                                n447 = local read "Stop"() -> (w516:bool)
                                n448 = And(x=w519, y=w520) -> (x .and. y?=w523:bool)
                                n449 = And(x=w517, y=w518) -> (x .and. y?=w524:bool)
                                n450 = And(x=w524, y=w523) -> (x .and. y?=w522:bool)
                                n451 = And(x=w522, y=w521) -> (x .and. y?=w525:bool)
                                n452 = Or(x=w527, y=w525) -> (x .or. y?=w526:bool)
                                n453 = Or(x=w526, y=w516) -> (x .or. y?=w515:bool)
                                }
                              }
                            }
                            n454 = local write "Calculate condition"(TRUE ("Calculate condition")) -> ()
                          }
                          frame #2 {
                            n455 = flat-sequence {
                              tunnel: w530 -> [w532]
                              tunnel: [w532] -> w529
                              tunnel: w529 -> [w536]
                              tunnel: [w536] -> w528
                              frame #0 {
                                n456 = local write "Equlibrating Temperature"(TRUE) -> ()
                              }
                              frame #1 {
                                # "Wait 1.5 system volumes"
                                n457 = local read "tau 2"() -> (w541:dbl)
                                n458 = local read "tau 4"() -> (w545:dbl)
                                n459 = local read "tau 3"() -> (w542:dbl)
                                n460 = local read "tau 5"() -> (w547:dbl)
                                n461 = local read "tau 1"() -> (w540:dbl)
                                n462 = Add(x=w540, y=w541) -> (x+y=w543:dbl)
                                n463 = Add(x=w543, y=w542) -> (x+y=w544:dbl)
                                n464 = Add(x=w544, y=w545) -> (x+y=w546:dbl)
                                n465 = Add(x=w546, y=w547) -> (x+y=w535:dbl)
                                n466 = Multiply(x=w535, y=2.0) -> (x*y=w533:dbl)
                                "Total System Resisdence Time(min)" <- w533
                                n467 = Multiply(x=w533, y=3) -> (x*y=w539:dbl)
                                "total_flush_time" <- w539
                                n468 = Multiply(x=60.0, y=w539) -> (x*y=w538:dbl)
                                n469 = property on="System Flush Wait Time" class="Slide (strict)"("Scale.Maximum"=w538) -> ()  [unwired: 2 in, 2 out]
                                n470 = script code="start = tic;"("total_wait_time"=w538) -> ("??"=w537:errorcluster)  [unwired: 1 in]
                                n471 = while {
                                tunnel: w536 -> [w551]
                                tunnel: w537 -> [w555]
                                stop <- w556 stop-if-true
                                # "Check if system is flushed every 10 seconds"
                                n472 = script code="end1 = toc(start);\nflush_time = 0;\nif end1 > 10\n   flush_time = 1;\nend\ncurr_wait_time = end1 /60;"("??"=w555) -> ("flush_time"=w559:dbl, "curr_wait_time"=w554:dbl)  [unwired: 1 out]
                                "curr_wait_time" <- w554
                                n473 = Not Equal To 0?(x=w559) -> (x != 0?=w558:bool)
                                n474 = Multiply(x=60.0, y=w554) -> (x*y=w553:dbl)
                                n475 = local read "Stop"() -> (w561:bool)
                                n476 = local write "System Flush Wait Time"(w553) -> ()
                                n477 = Or(x=w558, y=w561) -> (x .or. y?=w557:bool)
                                n478 = Not(x=w551) -> (.not. x?=w550:bool)
                                n479 = Wait (ms)(milliseconds to wait=u32 10000) -> ()  [unwired: 1 out]
                                n480 = Or(x=w557, y=w550) -> (x .or. y?=w556:bool)
                                }
                              }
                            }
                          }
                          frame #3 {
                            # "Collect HPLC Data"
                            n481 = local write "Flushing System"(TRUE ("Flushing System")) -> ()
                            n482 = flat-sequence {
                              tunnel: w563 -> [w570]
                              tunnel: w562 -> [w569]
                              frame #0 {
                                n483 = local read "pause for ms"() -> (w566:bool)
                                n484 = case shown="True" w566 {
                                frame False {
                                }
                                frame True {
                                n485 = One Button Dialog(message="Press OK to Analyze Data", button name ("OK")="OK" ("Left Button Text (\"Yes\")")) -> ()  [unwired: 1 out]
                                }
                                }
                              }
                              frame #1 {
                                n486 = flat-sequence {
                                tunnel: [w572] -> w571
                                tunnel: w571 -> [w578]
                                tunnel: w570 -> [w586]
                                tunnel: w569 -> [w587]
                                frame #0 {
                                n487 = disable-structure shown="Enabled" {
                                disable-tunnel: [w573 _] -> w572
                                frame Disabled {
                                n488 = local read "COMM Port :: Milligat Pumps"() -> (w574:refnum<visa-resource-name>)
                                n489 = local read "P_tot"() -> (w577:dbl)
                                n490 = Multiply(x=w577, y=2.0) -> (x*y=w573:dbl)
                                n491 = call "PumpDispense.vi"("Flowrate(ul/min)"=w573, "Pump Address"="f", "Pump COMM Port"=w574) -> ()  [unwired: 7 in, 2 out]
                                }
                                frame Enabled {
                                }
                                }
                                }
                                frame #1 {
                                n492 = disable-structure shown="Enabled" {
                                disable-tunnel: w578 -> [w580 _]
                                frame Disabled {
                                n493 = local read "Stop"() -> (w579:bool)
                                n494 = case shown="False" w579 {
                                tunnel: w580 -> [w581 _]
                                frame False {
                                n495 = Divide(x=400.0 ("y"), y=w581) -> (x/y=w583:dbl)
                                n496 = Multiply(x=60000.0, y=w583) -> (x*y=w585:dbl)
                                n497 = Wait (ms)(milliseconds to wait=w585) -> ()  [unwired: 1 out]
                                }
                                frame True {
                                }
                                }
                                }
                                frame Enabled {
                                }
                                }
                                }
                                frame #2 {
                                n498 = while {
                                tunnel: w586 -> [w597]
                                tunnel: w587 -> [w591]
                                tunnel: w586 -> [w588]
                                stop <- w592 stop-if-true
                                n499 = flat-sequence {
                                tunnel: w588 -> [w598]
                                tunnel: w597 -> [_]
                                tunnel: [w651] -> w590
                                tunnel: w590 -> [w659]
                                tunnel: [w666] -> w589
                                tunnel: [w668] -> w595
                                tunnel: w589 -> [w668]
                                frame #0 {
                                n500 = local read "COMM Port :: Milligat Pumps"() -> (w600:refnum<visa-resource-name>)
                                n501 = stacked-sequence {
                                tunnel: w600 -> [w603 w612 w621 w623 w629 w639]
                                tunnel: w598 -> [w602 w608 w618 w625 w631 w635]
                                tunnel: 1.0 ("Flowrate(ul/min)") -> [w601 w607 w616 w622 w628 w634]
                                frame #0 {
                                n502 = Index Array(array=w602, index=0) -> (element=w605:dbl)
                                n503 = Greater Than 0?(x=w605) -> (x > 0?=w604:bool)
                                n504 = case shown="True" w604 {
                                tunnel: w603 -> [_ _]
                                tunnel: w601 -> [_ _]
                                frame False {
                                }
                                frame True {
                                }
                                }
                                }
                                frame #1 {
                                n505 = Index Array(array=w608, index=1) -> (element=w610:dbl)
                                n506 = Greater Than 0?(x=w610) -> (x > 0?=w609:bool)
                                n507 = case shown="True" w609 {
                                tunnel: w607 -> [_ w614]
                                tunnel: w612 -> [_ w613]
                                frame False {
                                }
                                frame True {
                                n508 = local read "Syringe_pump?"() -> (w615:bool)
                                n509 = case shown="False" w615 {
                                tunnel: w614 -> [_ _]
                                tunnel: w613 -> [_ _]
                                frame False {
                                }
                                frame True {
                                }
                                }
                                }
                                }
                                }
                                frame #2 {
                                n510 = Index Array(array=w618, index=2) -> (element=w619:dbl)
                                n511 = Greater Than 0?(x=w619) -> (x > 0?=w617:bool)
                                n512 = case shown="True" w617 {
                                tunnel: w621 -> [_ _]
                                tunnel: w616 -> [_ _]
                                frame False {
                                }
                                frame True {
                                }
                                }
                                }
                                frame #3 {
                                n513 = Index Array(array=w625, index=3) -> (element=w626:dbl)
                                n514 = Greater Than 0?(x=w626) -> (x > 0?=w624:bool)
                                n515 = case shown="True" w624 {
                                tunnel: w623 -> [_ _]
                                tunnel: w622 -> [_ _]
                                frame False {
                                }
                                frame True {
                                }
                                }
                                }
                                frame #4 {
                                n516 = Index Array(array=w631, index=4) -> (element=w632:dbl)
                                n517 = Greater Than 0?(x=w632) -> (x > 0?=w630:bool)
                                n518 = case shown="True" w630 {
                                tunnel: w629 -> [_ _]
                                tunnel: w628 -> [_ _]
                                frame False {
                                }
                                frame True {
                                }
                                }
                                }
                                frame #5 {
                                n519 = Index Array(array=w635, index=5) -> (element=w637:dbl)
                                n520 = Greater Than 0?(x=w637) -> (x > 0?=w636:bool)
                                n521 = case shown="True" w636 {
                                tunnel: w639 -> [_ _]
                                tunnel: w634 -> [_ _]
                                frame False {
                                }
                                frame True {
                                }
                                }
                                }
                                }
                                }
                                frame #1 {
                                n522 = while {
                                stop <- w645 stop-if-true
                                n523 = local read "Phase_Sensor_voltage"() -> (w640:dbl)
                                n524 = script code="organic_phase = 0;\nif start_phase_time \n   start_phase_timer = tic;\n   start_phase_time = 0;\nelse\n  %ignore phase sensor values\n  %if not(phase_sensor_val >2.9 && phase_sensor_val <3.8)\n    %    start_phase_timer = tic;\n   %end\n\n   end_phase_time =  toc(start_phase_timer )\n\n   if end_phase_time > 2\n       organic_phase = 1;\n       start_phase_time = 1;\n   end\n\nend"("phase_sensor_val"=w640) -> ("organic_phase"=w642:dbl)  [unwired: 1 in, 1 out]
                                n525 = local read "Stop"() -> (w644:bool)
                                n526 = Not Equal To 0?(x=w642) -> (x != 0?=w643:bool)
                                n527 = Or(x=w643, y=w644) -> (x .or. y?=w645:bool)
                                n528 = Wait (ms)(milliseconds to wait=u32 300) -> ()  [unwired: 1 out]
                                }
                                }
                                frame #2 {
                                }
                                frame #3 {
                                n529 = Wait (ms)(milliseconds to wait=u32 2000) -> ()  [unwired: 1 out]
                                }
                                frame #4 {
                                }
                                frame #5 {
                                n530 = disable-structure shown="Enabled" {
                                frame Disabled {
                                n531 = local read "COMM Port :: Milligat Pumps"() -> (w647:refnum<visa-resource-name>)
                                n532 = call "PumpDispense.vi"("Flowrate(ul/min)"=10.0, "Pump Address"="f", "Pump COMM Port"=w647) -> ()  [unwired: 7 in, 2 out]
                                }
                                frame Enabled {
                                }
                                }
                                }
                                frame #6 {
                                }
                                frame #7 {
                                n533 = local read "Stop"() -> (w653:bool)
                                n534 = local read "Bay Parameters"() -> (w651:T3)
                                n535 = Unbundle By Name(w651) -> ("Hplc Wait time(min)"=w650:dbl)
                                n536 = Not(x=w653) -> (.not. x?=w652:bool)
                                n537 = case shown="True" w652 {
                                tunnel: w650 -> [_ w654]
                                frame False {
                                }
                                frame True {
                                # "Wait till for HPLC Method"
                                n538 = Multiply(x=u32 60000 ("milliseconds to wait"), y=w654) -> (x*y=w656:dbl)
                                n539 = Wait (ms)(milliseconds to wait=w656) -> ()  [unwired: 1 out]
                                }
                                }
                                }
                                frame #8 {
                                n540 = Unbundle By Name(w659) -> ("hplc File Name"=w660:string)
                                n541 = call "hplc_analyze.vi"("File Path"=w660) -> ("error out"=w658:errorcluster)  [unwired: 10 in]
                                n542 = Unbundle By Name(w658) -> ("status"=w657:bool)
                                n543 = case shown="True" w657 {
                                frame False {
                                }
                                frame True {
                                w661 = "An error occured while trying to read HPLC data. " ("message")
                                n544 = local write "Error Message"(w661) -> ()
                                n545 = Two Button Dialog(message=w661, 1:"STOP EXPs" ("F button name (\"Cancel\")"), 2:"REDO" ("T button name (\"OK\")")) -> (T button?=w662:bool)
                                n546 = case shown="True" w662 {
                                frame False {
                                w665 = TRUE ("Setup Error")
                                n547 = script code="system_error = 1"() -> ()  [unwired: 1 in, 1 out]
                                n548 = local write "Setup Error"(w665) -> ()
                                n549 = local write "Stop"(w665) -> ()
                                }
                                frame True {
                                n550 = script code="redo = true;"() -> ()  [unwired: 1 in, 1 out]
                                }
                                }
                                }
                                }
                                }
                                frame #9 {
                                n551 = script code="repeat = 0"() -> ("repeat"=w667:dbl)  [unwired: 1 in, 1 out]
                                n552 = Equal To 0?(x=w667) -> (x = 0?=w666:bool)
                                n553 = case shown="False" w666 {
                                frame False {
                                }
                                frame True {
                                }
                                }
                                }
                                frame #10 {
                                n554 = disable-structure shown="Disabled" {
                                frame Disabled {
                                n555 = flat-sequence {
                                tunnel: w670 -> [w675]
                                tunnel: [w675] -> _
                                tunnel: [w675] -> w669
                                frame #0 {
                                n556 = Wait (ms)(milliseconds to wait=u32 500) -> ()  [unwired: 1 out]
                                }
                                }
                                n557 = call-poly <vilib>:"Digital Write.vi"("Output Value"=FALSE, "DO Channel"=u8 22) -> ("LINX Resource"=w670:T10)  [unwired: 8 in, 1 out]
                                n558 = call-poly <vilib>:"Digital Write.vi"("Output Value"=TRUE, "DO Channel"=u8 22, "LINX Resource"=w669) -> ()  [unwired: 7 in, 2 out]
                                }
                                frame Enabled {
                                }
                                }
                                }
                                }
                                n559 = local read "Stop"() -> (w596:bool)
                                n560 = Not(x=w591) -> (.not. x?=w594:bool)
                                n561 = Or(x=w596, y=w595) -> (x .or. y?=w593:bool)
                                n562 = Or(x=w593, y=w594) -> (x .or. y?=w592:bool)
                                }
                                }
                                }
                              }
                              frame #2 {
                                n563 = script code="C_measured =P1/P2/T3*P3;\n%Fvalues(end +1,:) = [Conc];"() -> ()  [unwired: 1 in, 1 out]
                                n564 = local write "HPLC Analysis"(TRUE ("HPLC Analysis")) -> ()
                              }
                            }
                            "System Flushed?" <- TRUE ("System Flushed?")
                          }
                          frame #4 {
                            # "Save data to excel file"
                            n565 = local read "Total Number of Experiments"() -> (w678:dbl)
                            n566 = script code="if not(system_error) && not(redo)\n  if opt_ctr == 1\n        f(req_ctr,:) = [-(C_measured) sqrt(eps)];  \n     %f(req_ctr,:) = [-C_measured/total_wait_time sqrt(eps)];  \n  end\n  temp_write = [CurrExp, f(req_ctr,1), C_measured];\n  lastrowStr4 = num2str(lastrow4);\n  xlSheets.Item(idx4).Range(strcat('A',lastrowStr4,':',lastcol4,lastrowStr4)).Value2 =  temp_write;\n  lastrow4 = lastrow4 +1;\n  xlWorkbook.SaveAs(xl_file);\n  allHPLCData(end+1,:) =  [CurrExp new_x(:)' f(req_ctr,1) C_measured]\n  %allHPLCFile(end+1,:) = [num2str(CurrExp) hplc_file];\n\n  opt_ctr = 1;\n  CurrExp = CurrExp + 1;\n  terminate = 0;\n\n    if is_first_set_of_exp\n       ncall0 = size(f,1);\n       is_first_set_of_exp = false;\n    else\n       ncall0 = ncall0 +1;% size(f,1); % update function call counter\n    end\n    [fbestn,jbest] = min(f(:,1)); % best function value\n\n    if fbestn < fbest\n        fbest = fbestn;\n        xbest = x(jbest,:);\n        ncall0,xbest,fbest % display current number of function values,\n        % best point and function value if fbest has changed\n        nstop0 = 0;\n   \n    end\n  \n      % check stopping criterion\n    if nstop0 >= nstop  || ncall0 >= ncall\n       terminate = 1;\n       lastrowStr_temp = num2str(10);\n       lastcol_temp =  xlcolumnletter(length(xbest)+1);\n       xlSheets.Item(idx3).Range(strcat('B',lastrowStr_temp,':',lastcol_temp,lastrowStr_temp)).Value2 =  xbest;\n       xlWorkbook.SaveAs(xl_file);\n    end\n\n    if req_ctr == req_tot\n        if ncall >= minfcall && fbestn > fbest\n           nstop0 = nstop0 + 1;\n        end\n       opt_ctr = 3;\n    else\n       req_ctr = req_ctr +1;\n    end\n\n   save(matlabsavefile);\nend"("ncall"=w678) -> ("terminate"=w680:dbl, "ncall0"=w679:dbl)  [unwired: 1 in, 1 out]
                            n567 = local write "Current Experiment"(w679) -> ()
                          }
                          frame #5 {
                            n568 = local read "Num_exp_till_pause"() -> (w682:i32)
                            n569 = Increment(x=w682) -> (x+1=w681:i32)
                            n570 = local write "Num_exp_till_pause"(w681) -> ()
                          }
                          frame #6 {
                            # "Pause System"
                            n571 = local read "Bay Parameters"() -> (w690:T3)
                            n572 = Unbundle By Name(w690) -> ("Num_conditons_per_wait"=w689:dbl)
                            n573 = local read "Num_exp_till_pause"() -> (w688:i32)
                            n574 = Equal?(x=w689, y=w688) -> (x = y?=w687:bool)
                            n575 = local read "Run_Stop_cluster"() -> (w684:T6)
                            n576 = Unbundle By Name(w684) -> ("Stop Run Button"=w686:bool)
                            n577 = Or(x=w686, y=w687) -> (x .or. y?=w685:bool)
                            n578 = case shown="True" w685 {
                              tunnel: w689 -> [w693 _]
                              tunnel: w688 -> [w694 _]
                              tunnel: w684 -> [_ w696]
                              frame False {
                                n579 = Greater?(x=w694, y=w693) -> (0:w692:bool)
                                n580 = case shown="True" w692 {
                                frame False {
                                }
                                frame True {
                                n581 = local write "Num_exp_till_pause"(0 ("Num_exp_till_pause")) -> ()
                                }
                                }
                              }
                              frame True {
                                n582 = flat-sequence {
                                tunnel: w696 -> [w721]
                                frame #0 {
                                w700 = string[] ["e", "f", "g", "h", "i", "j"]
                                # "Turn off pumps and stop controling temperature"
                                n583 = stacked-sequence {
                                frame #0 {
                                n584 = local write "Temperature Control 1"(FALSE ("Temperature Control 1")) -> ()
                                }
                                frame #1 {
                                n585 = local write "Temperature Control 2"(FALSE ("Temperature Control 2")) -> ()
                                }
                                frame #2 {
                                n586 = local write "Temperature Control 3"(FALSE ("Temperature Control 3")) -> ()
                                }
                                frame #3 {
                                n587 = local write "Temperature Control 4"(FALSE ("Temperature Control 4")) -> ()
                                }
                                frame #4 {
                                n588 = local write "Temperature Control 5"(FALSE ("Temperature Control 5")) -> ()
                                }
                                }
                                n589 = local read "COMM Port:: Harvard Syringe Pump"() -> (w698:refnum<visa-resource-name>)
                                n590 = local read "Syringe_pump?"() -> (w697:bool)
                                n591 = local read "COMM Port :: Milligat Pumps"() -> (w699:refnum<visa-resource-name>)
                                n592 = Array Size(array=w700) -> (size(s)=w701:i32)
                                n593 = case shown="True" w697 {
                                tunnel: w698 -> [_ _]
                                frame False {
                                }
                                frame True {
                                }
                                }
                                n594 = for {
                                N: w701 -> [_]
                                tunnel: w700 -> [_] mode=indexing
                                tunnel: w699 -> [_]
                                }
                                }
                                frame #1 {
                                n595 = local read "Stop"() -> (w709:bool)
                                n596 = Not(x=w709) -> (.not. x?=w708:bool)
                                n597 = case shown="True" w708 {
                                frame False {
                                }
                                frame True {
                                n598 = while {
                                stop <- w715 stop-if-true
                                # "Wait till user confirms system resume"
                                n599 = Two Button Dialog(message="System is currently paused. Refill Syringes, flush lines, then press OK to continue optimization.\nOr Redo to repeat condition ", 1:"REDO" ("F button name (\"Cancel\")"), 2:"OK" ("Left Button Text (\"Yes\")")) -> (T button?=w711:bool)
                                n600 = case shown="False" w711 {
                                tunnel: [TRUE TRUE] -> w710
                                frame False {
                                n601 = script code="redo = true;"() -> ()  [unwired: 1 in, 1 out]
                                }
                                frame True {
                                }
                                }
                                n602 = local read "Stop"() -> (w716:bool)
                                n603 = Or(x=w710, y=w716) -> (x .or. y?=w715:bool)
                                }
                                }
                                }
                                n604 = local write "stop_xl_write"(TRUE ("stop_xl_write")) -> ()
                                }
                                frame #2 {
                                n605 = local write "Num_exp_till_pause"(0 ("Num_exp_till_pause")) -> ()
                                n606 = Bundle By Name(cluster=w721, "Stop Run Button"=FALSE) -> (w719:T6)
                                n607 = local write "Run_Stop_cluster"(w719) -> ()
                                }
                                }
                              }
                            }
                          }
                          frame #7 {
                            w724 = FALSE
                            n608 = local write "Equlibrating Temperature"(w724) -> ()
                            n609 = local write "Calculate condition"(w724) -> ()
                            n610 = local write "Flushing System"(w724) -> ()
                            n611 = local write "HPLC Analysis"(w724) -> ()
                            n612 = local write "stop_xl_write"(TRUE ("stop_xl_write")) -> ()
                          }
                        }
                        n613 = while {
                          stop <- w782 stop-if-true
                          n614 = flat-sequence {
                            frame #0 {
                              n615 = script code="temp_time_cond= [CurrExp, 1, P1, P2, P3, P4, P5,P6, T1, T2, T3, T4, T5, T1_SP, T2_SP, T3_SP, T4_SP, T5_SP, F1, F2, Pres1, Pres2];\n   lastrowStr1 = num2str(lastrow1);\n   xlSheets.Item(idx1).Range(strcat('A',lastrowStr1,':',lastcol1,lastrowStr1)).Value2 =   temp_time_cond;\n   lastrow1 = lastrow1+1;\n  xlWorkbook.SaveAs(xl_file);"() -> ()  [unwired: 1 in, 1 out]
                            }
                            frame #1 {
                              n616 = Wait (ms)(milliseconds to wait=u32 30000) -> ()  [unwired: 1 out]
                            }
                          }
                          n617 = local read "Stop"() -> (w783:bool)
                          n618 = local read "stop_xl_write"() -> (w781:bool)
                          n619 = Or(x=w781, y=w783) -> (x .or. y?=w782:bool)
                        }
                      }
                    }
                  }
                  frame True {
                    # "STANDBY MODE"
                    n620 = Add(x=w786, y=2.0) -> (x+y=w788:dbl)
                  }
                }
                n621 = Greater?(x=w373, y=w374) -> (0:w381:bool)
                n622 = Equal?(x=w379, y=1.0) -> (x = y?=w375:bool)
                n623 = local read "Stop"() -> (w382:bool)
                n624 = Or(x=w382, y=w381) -> (x .or. y?=w378:bool)
                n625 = Or(x=w375, y=w378) -> (x .or. y?=w377:bool)
                n626 = case shown="True" w375 {
                  frame False {
                  }
                  frame True {
                    n627 = local write "Stop"(TRUE ("Stop")) -> ()
                  }
                }
                "Optimization_loop_index" <- w383
              }
            }
          }
          n628 = while {
            stop <- w873 stop-if-true
            n629 = local read "Temperature Control 3"() -> (w869:bool)
            n630 = local read "Debug_run_button"() -> (w870:bool)
            n631 = Not(x=w870) -> (.not. x?=w872:bool)
            n632 = And(x=w872, y=w869) -> (x .and. y?=w871:bool)
            n633 = case shown="True" w871 {
              frame False {
                n634 = local write "Temp SS? 3"(TRUE) -> ()
              }
              frame True {
                # "Bay 3 Temperature Controller"
                n635 = local read "Temperature SP 3"() -> (w876:dbl)
                n636 = local read "Temperature 3"() -> (w879:dbl)
                n637 = Subtract(x=w879, y=w876) -> (x-y=w888:dbl)
                n638 = Absolute Value(x=w888) -> (abs(x)=w890:dbl)
                n639 = Less Or Equal?(x=w890, y=1.2) -> (x <= y?=w887:bool)
                n640 = local write "Temp SS? 3"(w887) -> ()
                n641 = local read "SSR Duration 3"() -> (w897:dbl)
                n642 = call-poly <vilib>:"PID Online Autotuning.vi"("setpoint"=w876, "manipulated variable"=w897, "autotuning parameters"=T8 {"type of controller"=enum."PID", "relay cycles"=3, "relay amplitude"=1.0, "control specifications"=enum."Normal", "PV noise level"=0.1} ("Autotuning Parameters R1"), "process variable"=w879, "PID gains in"=T7 {"Proportional gain Kc"=0.38538, "Integral time Ti (sec)"=0.524375, "Derivative time Ti (sec)"=0.12585} ("PID gains 2")) -> ("setpoint out"=w895:dbl, "process variable out"=w896:dbl, "PID gains out"=w899:T9)  [unwired: 6 in, 2 out]
                n643 = Greater?(x=w876, y=w879) -> (0:w886:bool)
                n644 = call <vilib>:"PID Autotuning (Temperature).vi"("desired temperature"=w895, "measured temperature"=w896, "PID gains in"=w899, "output range"=cluster{"output high":dbl, "output low":dbl} {"output high"=3.0, "output low"=-1.0} ("Output range")) -> ("output"=w892:dbl)  [unwired: 12 in, 3 out]
                n645 = Multiply(x=1000.0, y=w892) -> (x*y=w894:dbl)
                n646 = local write "SSR Duration 3"(w892) -> ()
                n647 = Greater Than 0?(x=w894) -> (x > 0?=w885:bool)
                n648 = And(x=w885, y=w886) -> (x .and. y?=w883:bool)
                n649 = Subtract(x=w879, y=10.0) -> (x-y=w881:dbl)
                n650 = Less?(x=w881, y=w876) -> (x < y?=w884:bool)
                n651 = And(x=w884, y=w883) -> (x .and. y?=w882:bool)
                n652 = case shown="False" w882 {
                  tunnel: 4 -> [_ _]
                  tunnel: w894 -> [w905 _]
                  tunnel: [0.0 w908] -> w877
                  tunnel: w876 -> [_ w907]
                  frame False {
                    (unwired) errorcluster {"status"=FALSE, "code"=0, "source"=""} ("error out")
                    n653 = Absolute Value(x=w905) -> (abs(x)=w906:dbl)
                    n654 = Wait (ms)(milliseconds to wait=w906) -> ()  [unwired: 1 out]
                  }
                  frame True {
                    n655 = script code="tempdiff3= SP3 - T3;\nif tempdiff3 > 10\n  if slope3 < .01\n     temp_check3 = temp_check3 + 1;\n  else\n      temp_check3 =0;\n  end\nend\n\nif temp_check3 > 9\n  temp_error3 = 1\nend"("SP3"=w907) -> ("temp_error3"=w908:dbl)  [unwired: 1 in, 1 out]
                  }
                }
                n656 = Not Equal To 0?(x=w877) -> (x != 0?=w878:bool)
                n657 = case shown="True" w878 {
                  frame False {
                  }
                  frame True {
                    n658 = local write "Error Message"("Bay 3 Temperature Heating Error") -> ()
                  }
                }
                n659 = case shown="True" w878 {
                  tunnel: w878 -> [_ w903]
                  frame False {
                  }
                  frame True {
                    n660 = local write "Stop"(w903) -> ()
                  }
                }
              }
            }
            n661 = Wait (ms)(milliseconds to wait=u32 400) -> ()  [unwired: 1 out]
            n662 = local read "Stop"() -> (w873:bool)
          }
          n663 = while {
            stop <- w833 stop-if-true
            n664 = local read "Debug_run_button"() -> (w829:bool)
            n665 = Not(x=w829) -> (.not. x?=w832:bool)
            n666 = Wait (ms)(milliseconds to wait=u32 400) -> ()  [unwired: 1 out]
            n667 = local read "Temperature Control 4"() -> (w831:bool)
            n668 = And(x=w832, y=w831) -> (x .and. y?=w830:bool)
            n669 = case shown="True" w830 {
              frame False {
                n670 = local write "Temp SS? 4"(TRUE ("Temp SS? 4")) -> ()
              }
              frame True {
                # "Bay 4 Temperature Controller"
                n671 = local read "Temperature SP 4"() -> (w838:dbl)
                n672 = local read "Temperature 4"() -> (w841:dbl)
                n673 = Subtract(x=w841, y=w838) -> (x-y=w848:dbl)
                n674 = Absolute Value(x=w848) -> (abs(x)=w850:dbl)
                n675 = Less Or Equal?(x=w850, y=1.2) -> (x <= y?=w847:bool)
                n676 = local write "Temp SS? 4"(w847) -> ()
                n677 = local read "SSR Duration 4"() -> (w851:dbl)
                n678 = call-poly <vilib>:"PID Online Autotuning.vi"("setpoint"=w838, "manipulated variable"=w851, "autotuning parameters"=T8 {"type of controller"=enum."PID", "relay cycles"=3, "relay amplitude"=1.0, "control specifications"=enum."Normal", "PV noise level"=0.1} ("Autotuning Parameters R1"), "process variable"=w841, "PID gains in"=T7 {"Proportional gain Kc"=0.38538, "Integral time Ti (sec)"=0.524375, "Derivative time Ti (sec)"=0.12585} ("PID gains 2")) -> ("setpoint out"=w853:dbl, "process variable out"=w854:dbl, "PID gains out"=w856:T9)  [unwired: 6 in, 2 out]
                n679 = call <vilib>:"PID Autotuning (Temperature).vi"("desired temperature"=w853, "measured temperature"=w854, "PID gains in"=w856, "output range"=cluster{"output high":dbl, "output low":dbl} {"output high"=3.0, "output low"=-1.0} ("Output range")) -> ("output"=w852:dbl)  [unwired: 12 in, 3 out]
                n680 = Subtract(x=w841, y=10.0) -> (x-y=w840:dbl)
                n681 = Less?(x=w840, y=w838) -> (x < y?=w842:bool)
                n682 = Multiply(x=1000.0, y=w852) -> (x*y=w860:dbl)
                n683 = Greater?(x=w838, y=w841) -> (0:w846:bool)
                n684 = Greater Than 0?(x=w860) -> (x > 0?=w845:bool)
                n685 = local write "SSR Duration 4"(w852) -> ()
                n686 = And(x=w845, y=w846) -> (x .and. y?=w844:bool)
                n687 = And(x=w842, y=w844) -> (x .and. y?=w843:bool)
                n688 = case shown="False" w843 {
                  tunnel: 5 -> [_ _]
                  tunnel: w860 -> [w865 _]
                  tunnel: w838 -> [_ w868]
                  tunnel: [0.0 w867] -> w837
                  frame False {
                    (unwired) errorcluster {"status"=FALSE, "code"=0, "source"=""} ("error out")
                    n689 = Absolute Value(x=w865) -> (abs(x)=w866:dbl)
                    n690 = Wait (ms)(milliseconds to wait=w866) -> ()  [unwired: 1 out]
                  }
                  frame True {
                    n691 = script code="tempdiff4= SP4 - T4;\nif tempdiff4 > 10\n  if slope4 < .01\n     temp_check4 = temp_check4 + 1;\n  else\n      temp_check4 =0;\n  end\nend\n\nif temp_check4 > 9\n  temp_error4 = 1\nend"("SP4"=w868) -> ("temp_error4"=w867:dbl)  [unwired: 1 in, 1 out]
                  }
                }
                n692 = Not Equal To 0?(x=w837) -> (x != 0?=w836:bool)
                n693 = case shown="True" w836 {
                  frame False {
                  }
                  frame True {
                    n694 = local write "Error Message"("Bay 4 Temperature Heating Error") -> ()
                  }
                }
                n695 = case shown="True" w836 {
                  tunnel: w836 -> [_ w863]
                  frame False {
                  }
                  frame True {
                    n696 = local write "Stop"(w863) -> ()
                  }
                }
              }
            }
            n697 = local read "Stop"() -> (w833:bool)
          }
          n698 = while {
            stop <- w369 stop-if-true
            n699 = script code="TempArr1=circshift(TempArr1,9);\nTempArr2=circshift(TempArr2,9);\nTempArr3=circshift(TempArr3,9);\nTempArr4=circshift(TempArr4,9);\nTempArr5=circshift(TempArr5,9);\n\nTempArr1(10)=T1;\nTempArr2(10)=T2;\nTempArr3(10)=T3;\nTempArr4(10)=T4;\nTempArr5(10)=T5;\n\n[slope1 temp] = polyfit([1,2,3,4,5,6,7,8,9,10]',TempArr1,1);\nslope1 = slope1(1);\n[slope2 temp] = polyfit([1,2,3,4,5,6,7,8,9,10]',TempArr2,1);\nslope2= slope2(1);\n[slope3 temp] = polyfit([1,2,3,4,5,6,7,8,9,10]',TempArr3,1);\nslope3 = slope3(1);\n[slope4 temp] = polyfit([1,2,3,4,5,6,7,8,9,10]',TempArr4,1);\nslope4 = slope4(1);\n[slope5 temp] = polyfit([1,2,3,4,5,6,7,8,9,10]',TempArr5,1);\nslope5 = slope5(1);"() -> ()  [unwired: 1 in, 1 out]
            n700 = Wait (ms)(milliseconds to wait=u32 600) -> ()  [unwired: 1 out]
            n701 = local read "Stop"() -> (w369:bool)
          }
          n702 = while {
            stop <- w794 stop-if-true
            n703 = local read "Debug_run_button"() -> (w791:bool)
            n704 = Not(x=w791) -> (.not. x?=w793:bool)
            n705 = local read "Temperature Control 5"() -> (w790:bool)
            n706 = And(x=w793, y=w790) -> (x .and. y?=w792:bool)
            n707 = case shown="True" w792 {
              frame False {
                n708 = local write "Temp SS? 5"(TRUE ("Temp SS? 5")) -> ()
              }
              frame True {
                # "Bay 5 Temperature Controller"
                n709 = local read "SSR Duration 5"() -> (w811:dbl)
                n710 = local read "Temperature SP 5"() -> (w797:dbl)
                n711 = local read "Temperature 5"() -> (w800:dbl)
                n712 = Subtract(x=w800, y=w797) -> (x-y=w808:dbl)
                n713 = Absolute Value(x=w808) -> (abs(x)=w810:dbl)
                n714 = Less Or Equal?(x=w810, y=1.2) -> (x <= y?=w807:bool)
                n715 = local write "Temp SS? 5"(w807) -> ()
                n716 = call-poly <vilib>:"PID Online Autotuning.vi"("setpoint"=w797, "manipulated variable"=w811, "autotuning parameters"=T8 {"type of controller"=enum."PID", "relay cycles"=3, "relay amplitude"=1.0, "control specifications"=enum."Normal", "PV noise level"=0.1} ("Autotuning Parameters R1"), "process variable"=w800, "PID gains in"=T7 {"Proportional gain Kc"=0.38538, "Integral time Ti (sec)"=0.524375, "Derivative time Ti (sec)"=0.12585} ("PID gains 2")) -> ("setpoint out"=w813:dbl, "process variable out"=w814:dbl, "PID gains out"=w816:T9)  [unwired: 6 in, 2 out]
                n717 = call <vilib>:"PID Autotuning (Temperature).vi"("desired temperature"=w813, "measured temperature"=w814, "PID gains in"=w816, "output range"=cluster{"output high":dbl, "output low":dbl} {"output high"=3.0, "output low"=-1.0} ("Output range")) -> ("output"=w812:dbl)  [unwired: 12 in, 3 out]
                n718 = Multiply(x=1000.0, y=w812) -> (x*y=w820:dbl)
                n719 = Greater?(x=w797, y=w800) -> (0:w805:bool)
                n720 = Greater Than 0?(x=w820) -> (x > 0?=w806:bool)
                n721 = local write "SSR Duration 5"(w812) -> ()
                n722 = And(x=w806, y=w805) -> (x .and. y?=w803:bool)
                n723 = Subtract(x=w800, y=10.0) -> (x-y=w801:dbl)
                n724 = Greater?(x=w801, y=w797) -> (0:w804:bool)
                n725 = And(x=w804, y=w803) -> (x .and. y?=w802:bool)
                n726 = case shown="False" w802 {
                  tunnel: 6 -> [_ _]
                  tunnel: w820 -> [w825 _]
                  tunnel: [0.0 w828] -> w798
                  tunnel: w797 -> [_ w827]
                  frame False {
                    (unwired) errorcluster {"status"=FALSE, "code"=0, "source"=""} ("error out")
                    n727 = Absolute Value(x=w825) -> (abs(x)=w826:dbl)
                    n728 = Wait (ms)(milliseconds to wait=w826) -> ()  [unwired: 1 out]
                  }
                  frame True {
                    n729 = script code="tempdiff5= SP5 - T5;\n\nif tempdiff5 > 10\n  if slope5 < .01\n     temp_check5 = temp_check5 + 1;\n  else\n      temp_check5 =0;\n  end\nend\n\nif temp_check5 >9\n  temp_error5 = 1\nend"("SP5"=w827) -> ("temp_error5"=w828:dbl)  [unwired: 1 in, 1 out]
                  }
                }
                n730 = Not Equal To 0?(x=w798) -> (x != 0?=w796:bool)
                n731 = case shown="True" w796 {
                  frame False {
                  }
                  frame True {
                    n732 = local write "Error Message"("Bay 5 Temperature Heating Error") -> ()
                  }
                }
                n733 = case shown="True" w796 {
                  tunnel: w796 -> [_ w823]
                  frame False {
                  }
                  frame True {
                    n734 = local write "Stop"(w823) -> ()
                  }
                }
              }
            }
            n735 = Wait (ms)(milliseconds to wait=u32 400) -> ()  [unwired: 1 out]
            n736 = local read "Stop"() -> (w794:bool)
          }
        }
      }
      n737 = while {
        tunnel: errorcluster {"status"=FALSE, "code"=0, "source"=""} ("error out") -> [w116]
        stop <- w127 stop-if-true
        # "Bay 5 Temperature Read"
        # "Bay 4 Temperature Read"
        # "Bay 3 Temperature Read"
        # "Bay 2 Temperature Read"
        # "Bay 1 Temperature Read"
        n738 = local read "Temperature SP 1"() -> (w117:dbl)
        n739 = local read "Stop"() -> (w127:bool)
        n740 = local write "error out"(w116) -> ()
        n741 = Unbundle By Name(w116) -> ("status"=w108:bool)
        n742 = call-poly <vilib>:"PID Control Input Filter.vi"("input"=w117) -> ("output"=w124:dbl)  [unwired: 4 in]
        n743 = case shown="True" w108 {
          tunnel: w124 -> [w136 _]
          tunnel: [w136 w137] -> w109
          frame False {
            n744 = local write "Temperature 1"(w136) -> ()
          }
          frame True {
            n745 = local read "Temperature 1"() -> (w137:dbl)
          }
        }
        n746 = flat-sequence {
          frame #0 {
            n747 = Wait (ms)(milliseconds to wait=u32 100) -> ()  [unwired: 1 out]
          }
        }
        n748 = local read "Temperature SP 2"() -> (w112:dbl)
        n749 = call-poly <vilib>:"PID Control Input Filter.vi"("input"=w112) -> ("output"=w123:dbl)  [unwired: 4 in]
        n750 = case shown="True" w108 {
          tunnel: w123 -> [w134 _]
          tunnel: [w134 w135] -> w122
          frame False {
            n751 = local write "Temperature 2"(w134) -> ()
          }
          frame True {
            n752 = local read "Temperature 2"() -> (w135:dbl)
          }
        }
        n753 = flat-sequence {
          frame #0 {
            n754 = Wait (ms)(milliseconds to wait=u32 100) -> ()  [unwired: 1 out]
          }
        }
        n755 = local read "Temperature SP 3"() -> (w115:dbl)
        n756 = call-poly <vilib>:"PID Control Input Filter.vi"("input"=w115) -> ("output"=w121:dbl)  [unwired: 4 in]
        n757 = case shown="False" w108 {
          tunnel: w121 -> [w132 _]
          tunnel: [w132 w133] -> w110
          frame False {
            n758 = local write "Temperature 3"(w132) -> ()
          }
          frame True {
            n759 = local read "Temperature 3"() -> (w133:dbl)
          }
        }
        n760 = flat-sequence {
          frame #0 {
            n761 = Wait (ms)(milliseconds to wait=u32 100) -> ()  [unwired: 1 out]
          }
        }
        n762 = local read "Temperature SP 4"() -> (w113:dbl)
        n763 = local read "Temperature SP 5"() -> (w111:dbl)
        n764 = call-poly <vilib>:"PID Control Input Filter.vi"("input"=w113) -> ("output"=w114:dbl)  [unwired: 4 in]
        n765 = case shown="True" w108 {
          tunnel: w114 -> [w130 _]
          tunnel: [w130 w131] -> w120
          frame False {
            n766 = local write "Temperature 4"(w130) -> ()
          }
          frame True {
            n767 = local read "Temperature 4"() -> (w131:dbl)
          }
        }
        n768 = flat-sequence {
          frame #0 {
            n769 = Wait (ms)(milliseconds to wait=u32 100) -> ()  [unwired: 1 out]
          }
        }
        n770 = flat-sequence {
          frame #0 {
            n771 = Wait (ms)(milliseconds to wait=u32 100) -> ()  [unwired: 1 out]
          }
        }
        n772 = call-poly <vilib>:"PID Control Input Filter.vi"("input"=w111) -> ("output"=w119:dbl)  [unwired: 4 in]
        n773 = Build Array(w109, w122, w110, w120, w119) -> (w126:dbl[])
        n774 = Array To Cluster(array=w126) -> (cluster=→"Teperature Chart":T5)
        n775 = case shown="False" w108 {
          tunnel: w119 -> [w128 _]
          tunnel: [w128 w129] -> w118
          frame False {
            n776 = local write "Temperature 5"(w128) -> ()
          }
          frame True {
            n777 = local read "Temperature 5"() -> (w129:dbl)
          }
        }
        n778 = script code="MATLAB script"("T1"=w109, "T2"=w122, "T3"=w110, "T4"=w120, "T5"=w118) -> ()  [unwired: 1 in, 1 out]
      }
      n779 = while {
        stop <- w59 stop-if-true
        n780 = local read "Pump setpoint(ul/min) 1"() -> (w62:dbl)
        n781 = local read "Pump setpoint(ul/min) 2"() -> (w58:dbl)
        n782 = local read "Pump setpoint(ul/min) 3"() -> (w57:dbl)
        n783 = local read "Pump setpoint(ul/min) 4"() -> (w56:dbl)
        n784 = local read "Pump setpoint(ul/min) 5"() -> (w55:dbl)
        n785 = local read "Pump setpoint(ul/min) 6"() -> (w54:dbl)
        n786 = Build Array(w62, w58, w57, w56, w55, w54) -> (w63:dbl[])
        n787 = Array To Cluster(array=w63) -> (cluster=→"Pump Setpoints Chart":T5)
        n788 = Wait (ms)(milliseconds to wait=u32 5000) -> ()  [unwired: 1 out]
        n789 = local read "Stop"() -> (w59:bool)
      }
      n790 = while {
        stop <- w53 stop-if-true
        w49 = 0
        n791 = Wait (ms)(milliseconds to wait=u32 300) -> ()  [unwired: 1 out]
        n792 = Build Array(w49) -> (w50:i32[])
        n793 = Array To Cluster(array=w50) -> (cluster=→"Phase Sensor Chart":T4)
        n794 = local read "Stop"() -> (w53:bool)
        "Phase_Sensor_voltage" <- w49
      }
      n795 = while {
        stop <- w103 stop-if-true
        w69 = 270
        w80 = 600
        w89 = 600
        w64 = 1
        # "Read Pressure and Flowrate"
        n796 = local read "Stop"() -> (w103:bool)
        n797 = call-poly <vilib>:"PID Control Input Filter.vi"("input"=w64) -> ("output"=w96:dbl)  [unwired: 4 in]
        n798 = call-poly <vilib>:"PID Control Input Filter.vi"("input"=w64) -> ("output"=w95:dbl)  [unwired: 4 in]
        n799 = call-poly <vilib>:"PID Control Input Filter.vi"("input"=w64) -> ("output"=w85:dbl)  [unwired: 4 in]
        n800 = call-poly <vilib>:"PID Control Input Filter.vi"("input"=w64) -> ("output"=w76:dbl)  [unwired: 4 in]
        n801 = Subtract(x=w85, y=0.065) -> (x-y=w86:dbl)
        n802 = Subtract(x=w76, y=0.065) -> (x-y=w77:dbl)
        n803 = Multiply(x=104.96 ("y"), y=w96) -> (x*y=w97:dbl)
        n804 = Multiply(x=104.96 ("y"), y=w95) -> (x*y=w100:dbl)
        n805 = Subtract(x=w97, y=24.077) -> (x-y=w67:dbl)
        n806 = Multiply(x=2, y=w89) -> (x*y=w91:i32)
        n807 = Divide(x=w91, y=3.3) -> (x/y=w87:dbl)
        n808 = Multiply(x=w86, y=w87) -> (x*y=w88:dbl)
        n809 = Subtract(x=w88, y=w89) -> (x-y=w71:dbl)
        n810 = Subtract(x=w100, y=24.077) -> (x-y=w68:dbl)
        n811 = Multiply(x=2, y=w80) -> (x*y=w82:i32)
        n812 = Divide(x=w82, y=3.3) -> (x/y=w78:dbl)
        n813 = Multiply(x=w77, y=w78) -> (x*y=w79:dbl)
        n814 = Subtract(x=w79, y=w80) -> (x-y=w70:dbl)
        n815 = Build Array(w71, w70) -> (w74:dbl[])
        n816 = Array To Cluster(array=w74) -> (cluster=→"Flowrate Chart":T5)
        n817 = Build Array(w68, w67) -> (w75:dbl[])
        n818 = local write "Flowrate Sensor 1"(w71) -> ()
        n819 = local write "Flowrate Sensor 2"(w70) -> ()
        n820 = local write "Pressure 1"(w68) -> ()
        n821 = local write "Pressure 2"(w67) -> ()
        n822 = Array To Cluster(array=w75) -> (cluster=→"Pressure Chart":T5)
        n823 = Wait (ms)(milliseconds to wait=u32 500) -> ()  [unwired: 1 out]
        n824 = script code="MATLAB script"("F1"=w71, "F2"=w70, "Pres1"=w68, "Pres2"=w67) -> ()  [unwired: 1 in, 1 out]
        n825 = Greater?(x=w67, y=w69) -> (0:w65:bool)
        n826 = Greater?(x=w68, y=w69) -> (0:w66:bool)
        n827 = case shown="False" w66 {
          frame False {
          }
          frame True {
            w107 = TRUE ("Stop")
            n828 = local write "System Error"(w107) -> ()
            n829 = local write "Stop"(w107) -> ()
            n830 = local write "Error Message"("Pressure Sensor 1 readings above 250psi") -> ()
            n831 = script code="system_error = 1;"() -> ()  [unwired: 1 in, 1 out]
          }
        }
        n832 = case shown="False" w65 {
          frame False {
          }
          frame True {
            w105 = TRUE ("Stop")
            n833 = local write "System Error"(w105) -> ()
            n834 = local write "Error Message"("Pressure Sensor 2 readings above 250psi") -> ()
            n835 = local write "Stop"(w105) -> ()
            n836 = script code="system_error = 1;"() -> ()  [unwired: 1 in, 1 out]
          }
        }
      }
    }
    frame #3 {
      # "Save and close xml and excel file"
      n837 = script code="if exist('xl_file','var') & exist('xlApp','var')\n  xlWorkbook.SaveAs(xl_file);\n  xlWorkbook.Close;\n  xlApp.Quit;\n  xlApp.delete;\nend"() -> ()  [unwired: 1 in, 1 out]
    }
    frame #4 {
      w996 = string[] ["e", "f", "g", "h", "i", "j"]
      # "End communication to hardware"
      n838 = local read "Syringe_pump?"() -> (w994:bool)
      n839 = local read "COMM Port:: Harvard Syringe Pump"() -> (w995:refnum<visa-resource-name>)
      n840 = local read "COMM Port :: Milligat Pumps"() -> (w998:refnum<visa-resource-name>)
      n841 = Array Size(array=w996) -> (size(s)=w997:i32)
      n842 = case shown="True" w994 {
        tunnel: w995 -> [_ _]
        frame False {
        }
        frame True {
        }
      }
      n843 = for {
        N: w997 -> [_]
        tunnel: w996 -> [_] mode=indexing
        tunnel: w998 -> [_]
        n844 = Wait (ms)(milliseconds to wait=u32 100) -> ()  [unwired: 1 out]
      }
    }
    frame #5 {
      # "Display Error Messages if necessary"
      n845 = local read "Error Message"() -> (w1000:string)
      n846 = One Button Dialog(message=w1000) -> ()  [unwired: 1 in, 1 out]
    }
  }
